vi "USO_GUI_rot_stg.vi"() -> ()   [LabVIEW 2014]
uses:
  <vilib>/Platform/TimedLoop/XDataNode/timing_clust.ctl
  <vilib>/Platform/TimedLoop/XDataNode/nitl_modes.ctl
  <vilib>/Platform/TimedLoop/XDataNode/wakeup.ctl
  gfitsio/cfitsio-bitpix.ctl
  <vilib>/platform/TimedLoop/XDataNode/XDataNode.xnode
  gfitsio/gfitsio.lvlib
  <vilib>/gmath/NI_Gmath.lvlib
  <userlib>/Newport ESP301/Newport ESP301.lvlib
  <vilib>/Platform/TimedLoop/XDataNode/XDNodeRunTimeDep.lvlib
panel:
  in  "initial absolute position":dbl=-33.5 min=-2000000000.0 max=2000000000.0 format="%.6f"
  out "Start time Array":timestamp[](array[timestamp])
  out "End time Array":timestamp[](array[timestamp])
  in  "Voltage-Retardance file path for lcvr2":path
  in  "Start observation session":bool
  out "LCVR closing\nvariable":T1(array[cluster])
  out "LCVR variable":T2
  out "Current Lcvr Temp":dbl
  out "volt set of lcvr 2":dbl[](array[numeric]) format="%_6g"
  out "volt set of lcvr 1":dbl[](array[numeric]) format="%_6g"
  in  "Voltage-Retardance file path for lcvr1":path
  in  "LCVR Set Temperature":dbl=21.0 min=10.0 max=50.0
  out "Buf no 2":bool
  out "Buf no 1":bool
  out "hout":u64
  in  "OpenStructureIn":T3={"Size"=88, "InterfaceType"=1, "Camera Number"=0, "CameraNumAtInterface"=0, "OpenFlags"=[], "OpenDWFlags"=[], "OpenPtrs"=[]} {"InterfaceType" items=["IEEE1394/FireWire", "IEEE1394/FireWire", "Matrox Helios CameraLink", "SiliconSoftware MicroEnableIII CL", "National Instruments CameraLink", "Gigabit Ethernet", "USB", "SiliconSoftware MicroEnable IV CL", "Reserved", "Reserved", "Generic CameraLink with CLSER.DLL"]}
  out "Buff_no 2":i16
  out "Buff_no1":i16
  in  "Close USO software":bool
  in  "spectroscopy/spectropolarimetry tab":enum32{"Spectroscopy", "Spectropolarimetry"}(tab) caption="Tab Control"
  in  "Slide":cluster{i32, i32}(slide)={16384, 0} scale=0.0..16400.0
  in  "Display Intensity control":bool
  in  "Control Pannel":T4
  in  "Cam Exp (msec)":dbl
  out "Cam Delay (msec)":dbl
  in  "Rot in deg":dbl min=-6000.0 max=6000.0 step=0.01
  in  "Scan steps":dbl=240.0
  out "Steps performed":i32(slide) max=190 scale=0.0..240.0
  in  "Start Spectroscopy":bool
  in  "Stop Spectroscopy":bool
  out "CCD Display":i32[][](graph)
  out "Data is stored in the folder.........":path
  in  "accept intensity":bool
  in  "Averaging \nNum":dbl=1.0
  in  "Image averaging":enum32{"Per scan", "Per Polarisation"}(radio)
  in  "LCVR Temperature in deg C\n      Set         Current":dbl[](array[numeric]) min=0.0 max=50.0
  in  "Slide sp":cluster{i32, i32}(slide)={16384, 0} scale=0.0..16400.0
  in  "accept intensity sp":bool
  out "Data is stored in the folder sp.........":path
  out "CCD Display sp":i32[][](graph)
  in  "Stop Spectroscopy sp":bool
  in  "Start Spectroscopy sp":bool
  out "Steps performed sp":i32(slide) max=190 scale=0.0..240.0
  in  "Scan steps sp":dbl=240.0
  in  "Rot in deg sp":dbl min=-6000.0 max=6000.0 step=0.01
  out "Cam Delay (msec) sp":dbl
  in  "Cam Exp (msec) sp":dbl
  in  "Display Intensity control sp":bool
  in  "Control Pannel sp":T4
  out "Motor Variable":T5={"VISA resource name"="", "Axis 2"=1, "Rotate in deg 2"=100.0, "Error In"={"status"=FALSE, "code"=0, "source"=""}}
  out "Cam Variable":T6
  in  "Rotate in deg":dbl=0.003
  in  "VISA Refnum in":refnum<visa-resource-name>
  in  "Axis":u32=1
  in  "CONTROLLER Number":string="1"
  out "Status":string
  in  "Apply":bool
  in  "InterfaceType":u32(ring)=6 items=["Ethernet"=5, "USB"=6]
  in  "Finish":bool
  out "Cam Detail":T7
  in  "Delay in msec":u32 max=4233600000
  in  "Exposure in msec":u32=30 min=500 max=4233600000
  in  "Initialise Device":u16(ring)=3 items=["Camera", "Liquid crystal", "Scan mirror", "--FF--"]
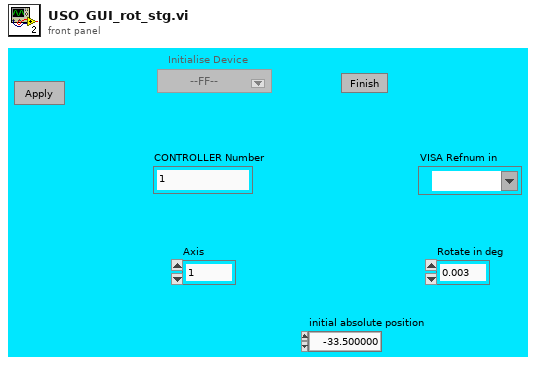
[diagram p1: front panel]
types:
  T1 = cluster{"Device Handle":u32, "Pipe 0 Handle":u32, "Pipe 1 Handle":u32}[]
  T2 = cluster{"Open USB I/O Stuff":cluster{"Device Handle":u32, "Pipe 0 Handle":u32, "Pipe 1 Handle":u32}, "volt set of lcvr 1":dbl[], "volt set of lcvr 2":dbl[], "LCVR Set Temperature":dbl, "Current Lcvr Temp":dbl}
  T3 = cluster{"Size":u16, "InterfaceType":u16, "Camera Number":u16, "CameraNumAtInterface":u16, "OpenFlags":u16[], "OpenDWFlags":u32[], "OpenPtrs":u32[]}
  T4 = cluster{"Move mirror":bool, "Preview":bool, "reset motor":bool, "motor home":bool, "Restore default values":bool}
  T5 = cluster{"VISA resource name":refnum<visa-resource-name>, "Axis 2":u32, "Rotate in deg 2":dbl, "Error In":errorcluster}
  T6 = cluster{"hout":u64, "ErrorOut":errorcluster, "Description":cluster{"Size":u16, "SensorTypeDESC":u16, "SensorSubtypeDESC":u16, "MaxHorizontalResStdDESC":u16, "MaxVerticalResStdDESC":u16, "MaxHorizontalResExtDESC":u16, "MaxVerticalResExtDESC":u16, "DynResDESC":u16, "MaxBinHorzDESC":u16, "BinHorzStepDESC":bool, "MaxBinVertDESC":u16, "BinVertStepDESC":bool, "ROIHorzStepDESC":u16, "ROIVertStepDESC":u16, "NumADCDESC":u16, "IRDESC":bool, "MinDelayDESC":u32, "MaxDelayDESC":u32, "MinDelayStepDESC":u32, "MinExpoDESC":u32, "MaxExpoDESC":u32, "MinExpoStepDESC":u32, "MinDelayIRDESC":u32, "MaxDelayIRDESC":u32, "MinExpoIRDESC":u32, "MaxExpoIRDESC":u32, "TimeTableDESC":bool, "DoubleImageDESC":bool, "MinCoolSetDESC":i16, "MaxCoolSetDESC":i16, "MDefaultCoolSetDESC":i16, "PowerDownModeDESC":bool, "OffsetRegDESC":bool, "ColorPattern":cluster{"UpperLeftColor":u8, "UpperRightColor":u8, "LowerLeftColor":u8, "LowerRightColor":u8}, "PatternTypeDESC":bool, "PixelRates":u32[], "CoversionFactors":u16[], "Reserved":u32[], "NoiseFilterCapable":bool, "HotPixelCapable":bool, "HotPixelWithNoiseFilter":bool, "ASCIITimeCapable":bool, "Extended Description":bool, "Get Extended":bool, "Reserved Flag 1":bool, "Reserved Flag 2":bool}}
  T7 = cluster{"Size":u16, "SensorTypeDESC":u16, "SensorSubtypeDESC":u16, "MaxHorizontalResStdDESC":u16, "MaxVerticalResStdDESC":u16, "MaxHorizontalResExtDESC":u16, "MaxVerticalResExtDESC":u16, "DynResDESC":u16, "MaxBinHorzDESC":u16, "BinHorzStepDESC":bool, "MaxBinVertDESC":u16, "BinVertStepDESC":bool, "ROIHorzStepDESC":u16, "ROIVertStepDESC":u16, "NumADCDESC":u16, "IRDESC":bool, "MinDelayDESC":u32, "MaxDelayDESC":u32, "MinDelayStepDESC":u32, "MinExpoDESC":u32, "MaxExpoDESC":u32, "MinExpoStepDESC":u32, "MinDelayIRDESC":u32, "MaxDelayIRDESC":u32, "MinExpoIRDESC":u32, "MaxExpoIRDESC":u32, "TimeTableDESC":bool, "DoubleImageDESC":bool, "MinCoolSetDESC":i16, "MaxCoolSetDESC":i16, "MDefaultCoolSetDESC":i16, "PowerDownModeDESC":bool, "OffsetRegDESC":bool, "ColorPattern":cluster{"UpperLeftColor":u8, "UpperRightColor":u8, "LowerLeftColor":u8, "LowerRightColor":u8}, "PatternTypeDESC":bool, "PixelRates":u32[], "CoversionFactors":u16[], "Reserved":u32[], "NoiseFilterCapable":bool, "HotPixelCapable":bool, "HotPixelWithNoiseFilter":bool, "ASCIITimeCapable":bool, "Extended Description":bool, "Get Extended":bool, "Reserved Flag 1":bool, "Reserved Flag 2":bool}
  T8 = enum16{"Find +0 Position Count", "Find Home and Index Signals", "Find Home Signal", "Find Positive Limit Signal", "Find Negative Limit Signal", "Find Positve Limit and Index Signals", "Find Negative Limit and Index Signals"}
  T9 = typedef "XDNodeRunTimeDep.lvlib/timing_clust.ctl" = cluster{"Expected End [f-1]":u64, "Actual End [f-1]":u64, "Finished Late? [f-1]":bool, "Expected End [i-1]":u64, "Actual End [i-1]":u64, "Finished Late? [i-1]":bool, "Expected Start [i]":u64, "Actual Start [i]":u64, "Expected Start [f]":u64, "Actual Start [f]":u64, "Source Name":string, "Structure Name":string, "Period":i64, "Deadline":i64, "Offset":i64, "Start":i64, "Priority":i32, "Timeout":i32, "Mode":T10, "Wakeup Reason":T11, "Error":errorcluster, "Source Type":string, "Secondary Source Type":string, "Global End Time":u64, "Global Start Time":u64, "Frame Duration":u64, "Iteration Duration":u64, "Assigned CPU":i32, "I/O Scan Engine Mode":u32}
  T10 = typedef "XDNodeRunTimeDep.lvlib/nitl_modes.ctl" = enum32{"No Change", "Process missed periods, maintain original phase", "Discard missed periods, maintain original phase", "Process missed periods, ignore original phase", "Discard missed periods, ignore original phase"}
  T11 = typedef "XDNodeRunTimeDep.lvlib/wakeup.ctl" = enum32{"Normal", "Aborted", "Asynchronous wakeup", "Timing source error", "Timed loop error", "Timeout"}
  T12 = enum8{"Enabled", "Disabled", "Disabled and Grayed Out"}
  T13 = enum16{"open", "open or create", "create or replace", "create", "open (read only)"}
  T14 = cluster{"Device Handle":u32, "Pipe 0 Handle":u32, "Pipe 1 Handle":u32}
  T15 = cluster{"Open USB I/O Stuff":cluster{"Device Handle":u32, "Pipe 0 Handle":u32, "Pipe 1 Handle":u32}, "yi":dbl[], "yi":dbl[], dbl, "Temp":dbl}
  T16 = cluster{"VISA resource name out":refnum<visa-resource-name>, "Axis":u32, "Rotate in deg":dbl, "error out":errorcluster}
  T17 = cluster{"hout":u64, "error out":errorcluster, "Description":cluster{"Size":u16, "SensorTypeDESC":u16, "SensorSubtypeDESC":u16, "MaxHorizontalResStdDESC":u16, "MaxVerticalResStdDESC":u16, "MaxHorizontalResExtDESC":u16, "MaxVerticalResExtDESC":u16, "DynResDESC":u16, "MaxBinHorzDESC":u16, "BinHorzStepDESC":bool, "MaxBinVertDESC":u16, "BinVertStepDESC":bool, "ROIHorzStepDESC":u16, "ROIVertStepDESC":u16, "NumADCDESC":u16, "IRDESC":bool, "MinDelayDESC":u32, "MaxDelayDESC":u32, "MinDelayStepDESC":u32, "MinExpoDESC":u32, "MaxExpoDESC":u32, "MinExpoStepDESC":u32, "MinDelayIRDESC":u32, "MaxDelayIRDESC":u32, "MinExpoIRDESC":u32, "MaxExpoIRDESC":u32, "TimeTableDESC":bool, "DoubleImageDESC":bool, "MinCoolSetDESC":i16, "MaxCoolSetDESC":i16, "MDefaultCoolSetDESC":i16, "PowerDownModeDESC":bool, "OffsetRegDESC":bool, "ColorPattern":cluster{"UpperLeftColor":u8, "UpperRightColor":u8, "LowerLeftColor":u8, "LowerRightColor":u8}, "PatternTypeDESC":bool, "PixelRates":u32[], "CoversionFactors":u16[], "Reserved":u32[], "NoiseFilterCapable":bool, "HotPixelCapable":bool, "HotPixelWithNoiseFilter":bool, "ASCIITimeCapable":bool, "Extended Description":bool, "Get Extended":bool, "Reserved Flag 1":bool, "Reserved Flag 2":bool}}
  T18 = typedef "gfitsio.lvlib/cfitsio-bitpix.ctl" = i32
  T19 = typedef "gfitsio.lvlib/gfitsio-refnum.ctl" = refnum<k1>
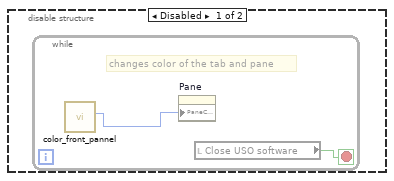
[diagram p2: hidden frame]
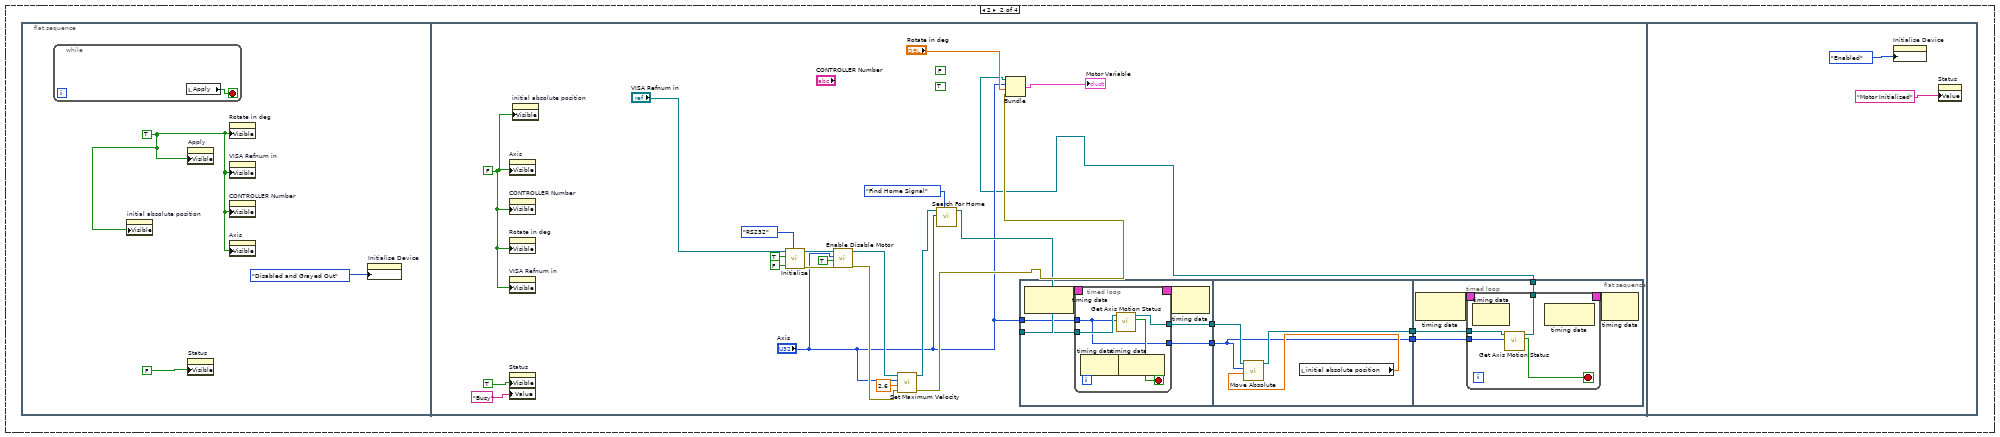
[diagram p9: hidden frame]
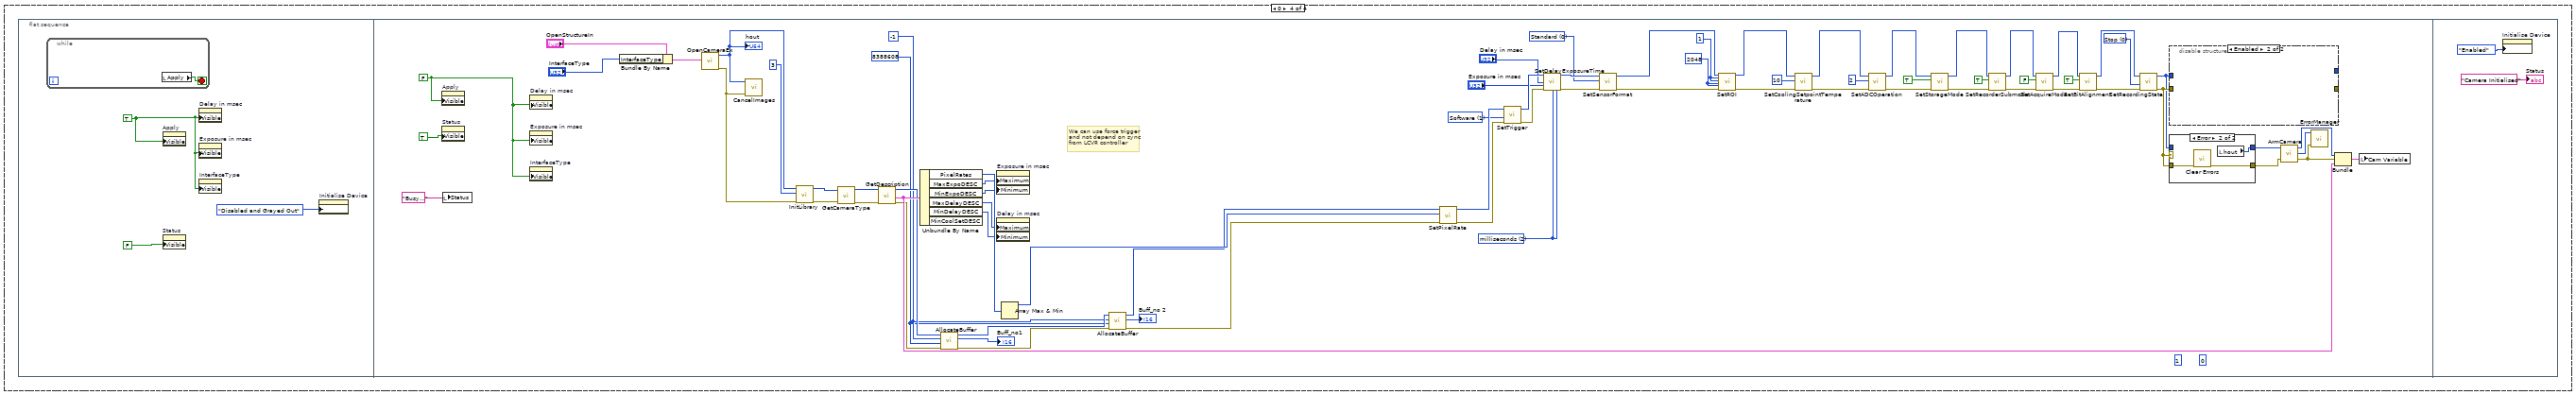
[diagram p11: hidden frame]
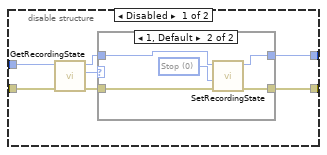
[diagram p12: hidden frame]
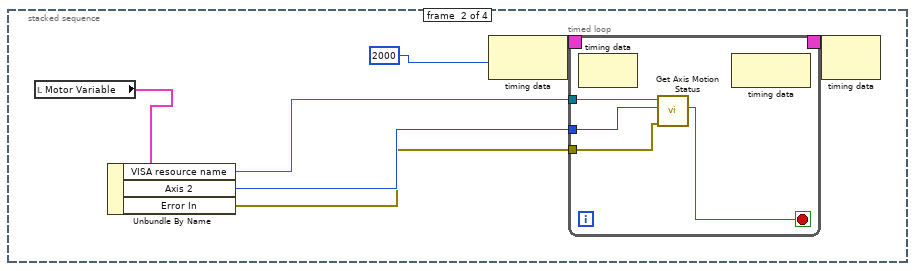
[diagram p15: hidden frame]
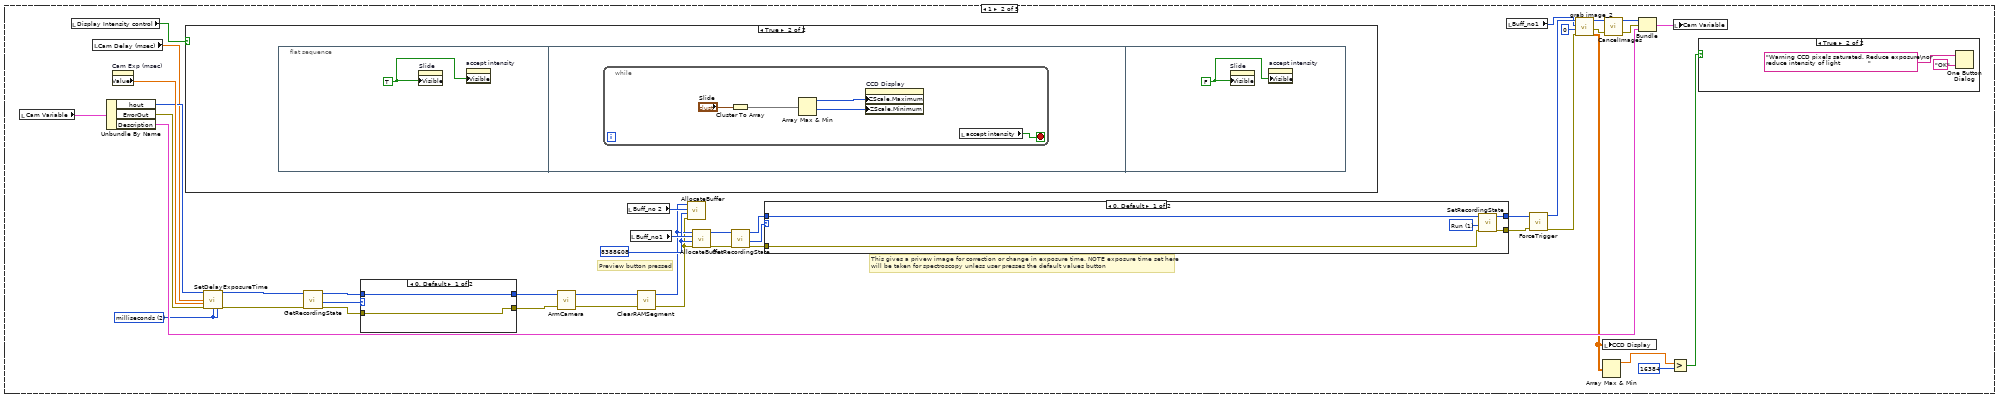
[diagram p18: hidden frame]
diagram:
  w2 = TRUE
  w3 = 2048.0 ("X Scale.Range:Maximum")
  w4 = 1.0 ("X Scale.Range:Minimum")
  w1 = FALSE
  # "Frame 0:- Initialize camera, lcvr, rotation stage\nFrame 1:- wait for rotation stage to complete roration (This is jst a safty measure, the code by default goes to frame 1 after completly initializing all components in frame 0 \n                  but a redundant frame is used for rotation stage jst to ensure completion of rotation stage's initialization)\nFrame 2:- The entire code runs in frame 2 right from previews, motor moves, frame recording, intensity range variation of image display,polcal, flat field  etc\nFrame 3:- Closes camera and LCVR and brings motor to home position and switches off the motor"
  n1 = disable-structure shown="Enabled" {
    frame Disabled {
      n2 = while {
        stop <- w6 stop-if-true
        # "changes color of the tab and pane"
        n3 = call "color_front_pannel.vi"() -> ("Resolved Color"=w5:u32)  [unwired: 11 in]
        n4 = property on="Pane" class="Pane"("PaneColor"=w5) -> ()  [unwired: 2 in, 2 out]
        n5 = local read "Close USO software"() -> (w6:bool)
      }
    }
    frame Enabled {
    }
  }
  n6 = stacked-sequence {
    frame #0 {
      n7 = Two Button Dialog(message="Initialise Devices ?", 1:"No" ("F button name (\"Cancel\")"), 2:"Yes" ("T button name (\"OK\")")) -> (T button?=w7:bool)
      n8 = case shown="True" w7 {
        frame False {
          n9 = flat-sequence {
            frame #0 {
              w11 = TRUE
              n10 = property on="Voltage-Retardance file path for lcvr2" class="Path"("Visible"=w11) -> ()  [unwired: 2 in, 2 out]
              n11 = property on="Voltage-Retardance file path for lcvr1" class="Path"("Visible"=w11) -> ()  [unwired: 2 in, 2 out]
              n12 = property on="initial absolute position" class="DigNum (strict)"("Visible"=w11) -> ()  [unwired: 2 in, 2 out]
              n13 = while {
                stop <- w12 stop-if-true
                n14 = local read "Apply"() -> (w12:bool)
              }
              n15 = property on="Apply" class="Bool (strict)"("Visible"=w11) -> ()  [unwired: 2 in, 2 out]
            }
            frame #1 {
              w17 = 1 ("Axis (1)")
              w14 = FALSE
              w52 = 21.0
              w69 = u32 8388608 ("Size")
              w70 = i16 -1 ("BufNr")
              w77 = u16 0 items=["Stop", "Run"] ("RecordingState")
              # "Dont use Arm Cam.vi here coz the camera FPGA \"remembers\"\nthe settings that were used in its previous use. So the camera \nwill be initialized to those settings automatically"
              # "As the user has not selected device initilization, all devices will be initiated to their default value"
              n16 = local read "Voltage-Retardance file path for lcvr2"() -> (w38:path)
              n17 = local read "Voltage-Retardance file path for lcvr1"() -> (w39:path)
              n18 = property on="Apply" class="Bool (strict)"("Visible"=w14) -> ()  [unwired: 2 in, 2 out]
              n19 = property on="Voltage-Retardance file path for lcvr2" class="Path"("Visible"=w14) -> ()  [unwired: 2 in, 2 out]
              n20 = property on="initial absolute position" class="DigNum (strict)"("Visible"=w14) -> ()  [unwired: 2 in, 2 out]
              n21 = property on="Voltage-Retardance file path for lcvr1" class="Path"("Visible"=w14) -> ()  [unwired: 2 in, 2 out]
              n22 = call "Meadowlark USB Easy Open.vi"() -> ("USB Device and Pipes Array"=w47:T1, "Device Count"=w13:u32)  [unwired: 1 out]
              n23 = case shown="0" w13 {
                frame 0 {
                  n24 = One Button Dialog(message="WARNING !!\nNO LCVR'S DETECTED", button name ("OK")="OK") -> ()  [unwired: 1 out]
                }
                frame 1, Default {
                }
              }
              n25 = call "volt vs retardance.vi"("file path (dialog if empty)"=w38) -> ("retardance in degree(known)"=w40:dbl[], "Voltage(unknown)"=w41:dbl[])  [unwired: 9 in]
              n26 = local write "LCVR closing\nvariable"(w47) -> ()
              n27 = local read "OpenStructureIn"() -> (w64:T3)
              n28 = call "volt vs retardance.vi"("file path (dialog if empty)"=w39) -> ("retardance in degree(known)"=w57:dbl[], "Voltage(unknown)"=w56:dbl[])  [unwired: 9 in]
              n29 = Index Array(array=w47, index=0) -> (element=w53:T14)
              n30 = local read "VISA Refnum in"() -> (w37:refnum<visa-resource-name>)
              n31 = local read "InterfaceType"() -> (w62:u32)
              n32 = call "Set temp.vi"("Temp"=w52, "USB Open Device Cluster"=w53) -> ()  [unwired: 1 in]
              n33 = call <vilib>:"Spline Interpolation 1D.vi"("xi"=dbl[] [45.0, 135.0, 135.0, 225.0], "X"=w57, "Y"=w56) -> ("yi"=w50:dbl[])  [unwired: 6 in, 2 out]
              n34 = call "read temp.vi"("USB Open Device Cluster"=w53) -> ("Temp"=w51:dbl)
              n35 = call <vilib>:"Spline Interpolation 1D.vi"("xi"=dbl[] [54.74, 125.26, 234.74, 54.74], "X"=w40, "Y"=w41) -> ("yi"=w49:dbl[])  [unwired: 6 in, 2 out]
              n36 = local write "LCVR Set Temperature"(w52) -> ()
              n37 = local write "Current Lcvr Temp"(w51) -> ()
              n38 = Bundle By Name(cluster=w64, "InterfaceType"=w62) -> (w61:T3)
              n39 = local write "volt set of lcvr 1"(w50) -> ()
              n40 = local write "volt set of lcvr 2"(w49) -> ()
              n41 = Bundle("Open USB I/O Stuff"=w53, "yi"=w50, "yi"=w49, w52, "Temp"=w51) -> (w48:T15)  [unwired: 1 in]
              n42 = local write "LCVR variable"(w48) -> ()
              n43 = call <userlib>:"OpenCameraEx.vi"("OpenStructureIn"=w61) -> ("error out"=w59:errorcluster, "hout"=w60:u64)  [unwired: 3 in, 2 out]
              n44 = call <userlib>:"CancelImages.vi"("error in (no error)"=w59, "ph"=w60) -> ()  [unwired: 1 in, 3 out]
              n45 = call <userlib>:"Initialize.vi"("VISA resource name"=w37, "ID Query (True)"=TRUE, "Reset (False)"=FALSE, "Serial Link (RS232)"=enum16{"RS232", "USB"}."RS232") -> ("VISA resource name out"=w33:refnum<visa-resource-name>, "error out"=w31:errorcluster)  [unwired: 5 in]
              n46 = call <userlib>:"InitLibrary.vi"("error in (no error)"=w59, "InterfaceType"=u32 3, "ph"=w60) -> ("error out"=w83:errorcluster, "hout"=w84:u64)  [unwired: 7 in]
              n47 = local read "Rotate in deg"() -> (w78:dbl)
              n48 = call <userlib>:"GetCameraType.vi"("ph"=w84, "error in (no error)"=w83) -> ("hout"=w82:u64, "error out"=w81:errorcluster)  [unwired: 1 in, 2 out]
              n49 = local read "Axis"() -> (w30:u32)
              n50 = call <userlib>:"Enable Disable Motor.vi"("error in (no error)"=w31, "Action (F - OFF)"=TRUE, "Axis (1)"=w17, "VISA resource name"=w33) -> ("error out"=w24:errorcluster, "VISA resource name out"=w26:refnum<visa-resource-name>)  [unwired: 2 in]
              n51 = call <userlib>:"GetDescription.vi"("ErrorIn"=w81, "ph"=w82) -> ("ErrorOut"=w43:errorcluster, "Description"=w80:T7, "hout"=w45:u64)  [unwired: 2 in, 1 out]
              n52 = local write "Cam Detail"(w80) -> ()
              n53 = call <userlib>:"Set Maximum Velocity.vi"("error in (no error)"=w24, "Maximum Velocity (0 units/s)"=2.6, "Axis (1)"=w17, "VISA resource name"=w26) -> ("error out"=w22:errorcluster, "VISA resource name out"=w23:refnum<visa-resource-name>)  [unwired: 2 in]
              n54 = call <userlib>:"SetBitAlignment.vi"("error in (no error)"=w43, "BitAlignent"=TRUE, "ph"=w45) -> ("error out"=w42:errorcluster, "hout"=w44:u64)  [unwired: 2 in, 1 out]
              n55 = call <userlib>:"Search For Home.vi"("Home mode"=T8."Find Home Signal", "error in (no error)"=w22, "Axis (1)"=w17, "VISA resource name"=w23) -> ("error out"=w27:errorcluster, "VISA resource name out"=w16:refnum<visa-resource-name>)  [unwired: 3 in]
              n56 = Bundle("VISA resource name out"=w15, "Axis"=w30, "Rotate in deg"=w78, "error out"=w27) -> (w29:T16)  [unwired: 1 in]
              n57 = call <userlib>:"SetRecordingState.vi"("ErrorIn"=w42, "RecordingState"=w77, "ph"=w44) -> ("ErrorOut"=w65:errorcluster, "hout"=w66:u64)  [unwired: 2 in, 1 out]
              n58 = call <userlib>:"ErrorManager.vi"("ErrorIn"=w65, "ErrorCode"=w66) -> ()  [unwired: 3 in, 1 out]
              n59 = flat-sequence {
                tunnel: w16 -> [w90]
                tunnel: w17 -> [w89]
                tunnel: [w88] -> w21
                tunnel: [w87] -> w20
                tunnel: w21 -> [w104]
                tunnel: w20 -> [w101]
                tunnel: [w102] -> w19
                tunnel: [w101] -> w18
                tunnel: w19 -> [w107]
                tunnel: w18 -> [w106]
                tunnel: [w105] -> w15
                frame #0 {
                  n60 = node-c288() -> (w92:T9)  [unwired: 1 in]
                  n61 = timed-loop {
                    timing: w92 -> [_]
                    timing-out: [_] -> w91
                    tunnel: w90 -> [w96]
                    tunnel: w89 -> [w93]
                    tunnel: [w95] -> w88
                    tunnel: [w93] -> w87
                    stop <- w94 stop-if-true
                    n62 = node-c288() -> ()  [unwired: 1 in, 1 out]
                    n63 = node-c288() -> ()  [unwired: 1 in, 1 out]
                    n64 = call <userlib>:"Get Axis Motion Status.vi"("Axis (1)"=w93, "VISA resource name"=w96) -> ("Motion Done"=w94:bool, "VISA resource name out"=w95:refnum<visa-resource-name>)  [unwired: 3 in, 1 out]
                  }
                  n65 = node-c288(w91) -> ()  [unwired: 1 out]
                }
                frame #1 {
                  n66 = local read "initial absolute position"() -> (w103:dbl)
                  n67 = call <userlib>:"Move Absolute.vi"("Position (0 units)"=w103, "Axis (1)"=w101, "VISA resource name"=w104) -> ("VISA resource name out"=w102:refnum<visa-resource-name>)  [unwired: 3 in, 1 out]
                }
                frame #2 {
                  n68 = node-c288() -> (w109:T9)  [unwired: 1 in]
                  n69 = timed-loop {
                    timing: w109 -> [_]
                    timing-out: [_] -> w108
                    tunnel: w107 -> [w113]
                    tunnel: w106 -> [w112]
                    tunnel: [w111] -> w105
                    stop <- w110 stop-if-true
                    n70 = node-c288() -> ()  [unwired: 1 in, 1 out]
                    n71 = call <userlib>:"Get Axis Motion Status.vi"("Axis (1)"=w112, "VISA resource name"=w113) -> ("Motion Done"=w110:bool, "VISA resource name out"=w111:refnum<visa-resource-name>)  [unwired: 3 in, 1 out]
                    n72 = node-c288() -> ()  [unwired: 1 in, 1 out]
                  }
                  n73 = node-c288(w108) -> ()  [unwired: 1 out]
                }
              }
              n74 = case shown="Error" w65 {
                tunnel: [w119 w121] -> w73
                tunnel: w65 -> [w119 w122]
                tunnel: w66 -> [w118 _]
                tunnel: [w118 w120] -> w76
                tunnel: w45 -> [_ w120]
                frame No Error {
                }
                frame Error {
                  n75 = call <vilib>:"Clear Errors.vi"("error in (no error)"=w122) -> ("error out"=w121:errorcluster)  [unwired: 5 in, 1 out]
                }
              }
              n76 = local write "Motor Variable"(w29) -> ()
              n77 = call <userlib>:"AllocateBuffer.vi"("error in (no error)"=w73, "Size"=w69, "BufNr"=w70, "ph"=w76) -> ("error out"=w72:errorcluster, "BufNrOut"=w68:i16, "hout"=w75:u64)  [unwired: 2 in, 3 out]
              n78 = local write "Buff_no1"(w68) -> ()
              n79 = call <userlib>:"AllocateBuffer.vi"("error in (no error)"=w72, "Size"=w69, "BufNr"=w70, "ph"=w75) -> ("error out"=w71:errorcluster, "BufNrOut"=w67:i16, "hout"=w74:u64)  [unwired: 2 in, 3 out]
              n80 = Bundle("hout"=w74, "error out"=w71, "Description"=w80) -> (→"Cam Variable":T17)  [unwired: 1 in]
              n81 = local write "Buff_no 2"(w67) -> ()
            }
          }
        }
        frame True {
          n82 = flat-sequence {
            frame #0 {
              w124 = TRUE
              n83 = property on="Finish" class="Bool"("Visible"=w124) -> ()  [unwired: 2 in, 2 out]
              n84 = property on="Initialise Device" class="Ring (strict)"("DisabledEnum"=T12."Enabled" ("Disabled")) -> ()  [unwired: 2 in, 2 out]
              n85 = property on="Initialise Device" class="Ring (strict)"("Visible"=w124) -> ()  [unwired: 2 in, 2 out]
            }
            frame #1 {
              n86 = while {
                stop <- w126 stop-if-true
                n87 = event shown="[0] \"Finish\", \"Initialise Device\": Value Change" {
                  selector: _ -> [_]
                  dyn-events: _ -> [_]
                  timeout: _ -> [_]
                  tunnel: ["Finish"] -> w126
                  tunnel: [w128] -> w125
                  event "Finish", "Initialise Device": Value Change {
                    n88 = event-data() -> ()  [unwired: 1 in, 1 out]
                    n89 = case shown="True" "Finish" {
                      tunnel: [w130 3] -> w128
                      tunnel: "Initialise Device" -> [w130 _]
                      frame False {
                      }
                      frame True {
                      }
                    }
                  }
                }
                n90 = case shown="1" w125 {
                  frame 1 {
                    n91 = flat-sequence {
                      frame #0 {
                        w132 = TRUE ("Visible")
                        n92 = while {
                          stop <- w136 stop-if-true
                          n93 = local read "Apply"() -> (w136:bool)
                        }
                        n94 = property on="Voltage-Retardance file path for lcvr2" class="Path"("Visible"=w132) -> ()  [unwired: 2 in, 2 out]
                        n95 = property on="Apply" class="Bool (strict)"("Visible"=TRUE) -> ()  [unwired: 2 in, 2 out]
                        n96 = property on="Voltage-Retardance file path for lcvr1" class="Path"("Visible"=w132) -> ()  [unwired: 2 in, 2 out]
                        n97 = property on="LCVR Set Temperature" class="DigNum (strict)"("Visible"=w132) -> ()  [unwired: 2 in, 2 out]
                        n98 = property on="Status" class="Str"("Visible"=FALSE) -> ()  [unwired: 2 in, 2 out]
                        n99 = property on="Initialise Device" class="Ring (strict)"("DisabledEnum"=T12."Disabled and Grayed Out" ("Disabled")) -> ()  [unwired: 2 in, 2 out]
                      }
                      frame #1 {
                        w140 = FALSE ("Visible")
                        n100 = property on="Apply" class="Bool (strict)"("Visible"=w140) -> ()  [unwired: 2 in, 2 out]
                        n101 = property on="Status" class="Str"("Visible"=TRUE) -> ()  [unwired: 2 in, 2 out]
                        n102 = local write "Status"("Busy...." ("Status")) -> ()
                        n103 = property on="Voltage-Retardance file path for lcvr2" class="Path"("Visible"=w140) -> ()  [unwired: 2 in, 2 out]
                        n104 = property on="Voltage-Retardance file path for lcvr1" class="Path"("Visible"=w140) -> ()  [unwired: 2 in, 2 out]
                        n105 = property on="LCVR Set Temperature" class="DigNum (strict)"("Visible"=w140) -> ()  [unwired: 2 in, 2 out]
                        n106 = call "Meadowlark USB Easy Open.vi"() -> ("USB Device and Pipes Array"=w139:T1, "Device Count"=w137:u32)  [unwired: 1 out]
                        n107 = case shown="0" w137 {
                          frame 0 {
                            n108 = One Button Dialog(message="WARNING !!\nNO LCVR'S DETECTED", button name ("OK")="OK") -> ()  [unwired: 1 out]
                          }
                          frame 1, Default {
                          }
                        }
                        n109 = local read "Current Lcvr Temp"() -> (w145:dbl)
                        n110 = local read "volt set of lcvr 1"() -> (w147:dbl[])
                        n111 = local read "volt set of lcvr 2"() -> (w148:dbl[])
                        n112 = local write "LCVR closing\nvariable"(w139) -> ()
                        n113 = call "volt vs retardance.vi"("file path (dialog if empty)"="Voltage-Retardance file path for lcvr2") -> ("retardance in degree(known)"=w142:dbl[], "Voltage(unknown)"=w143:dbl[])  [unwired: 9 in]
                        n114 = Index Array(array=w139, index=0) -> (element=w138:T14)
                        n115 = call "Set temp.vi"("Temp"="LCVR Set Temperature", "USB Open Device Cluster"=w138) -> ()  [unwired: 1 in]
                        n116 = call "read temp.vi"("USB Open Device Cluster"=w138) -> ("Temp"=→"Current Lcvr Temp":dbl)
                        n117 = Bundle("Open USB I/O Stuff"=w138, "volt set of lcvr 1"=w147, "volt set of lcvr 2"=w148, "LCVR Set Temperature"="LCVR Set Temperature", "Current Lcvr Temp"=w145) -> (w144:T2)  [unwired: 1 in]
                        n118 = call "volt vs retardance.vi"("file path (dialog if empty)"="Voltage-Retardance file path for lcvr1") -> ("retardance in degree(known)"=w158:dbl[], "Voltage(unknown)"=w157:dbl[])  [unwired: 9 in]
                        n119 = local write "LCVR variable"(w144) -> ()
                        n120 = call <vilib>:"Spline Interpolation 1D.vi"("xi"=dbl[] [45.0, 135.0, 135.0, 225.0], "X"=w158, "Y"=w157) -> ("yi"=→"volt set of lcvr 1":dbl[])  [unwired: 6 in, 2 out]
                        n121 = call <vilib>:"Spline Interpolation 1D.vi"("xi"=dbl[] [54.74, 125.26, 234.74, 54.74], "X"=w142, "Y"=w143) -> ("yi"=→"volt set of lcvr 2":dbl[])  [unwired: 6 in, 2 out]
                      }
                      frame #2 {
                        n122 = property on="Initialise Device" class="Ring (strict)"("DisabledEnum"=T12."Enabled" ("Disabled")) -> ()  [unwired: 2 in, 2 out]
                        n123 = local write "Status"("LCVR Initialised" ("Status")) -> ()
                      }
                    }
                  }
                  frame 2 {
                    n124 = flat-sequence {
                      frame #0 {
                        w164 = TRUE
                        n125 = while {
                          stop <- w167 stop-if-true
                          n126 = local read "Apply"() -> (w167:bool)
                        }
                        n127 = property on="initial absolute position" class="DigNum (strict)"("Visible"=w164) -> ()  [unwired: 2 in, 2 out]
                        n128 = property on="Apply" class="Bool (strict)"("Visible"=w164) -> ()  [unwired: 2 in, 2 out]
                        n129 = property on="Status" class="Str"("Visible"=FALSE) -> ()  [unwired: 2 in, 2 out]
                        n130 = property on="Rotate in deg" class="DigNum (strict)"("Visible"=w164) -> ()  [unwired: 2 in, 2 out]
                        n131 = property on="VISA Refnum in" class="VISAName"("Visible"=w164) -> ()  [unwired: 2 in, 2 out]
                        n132 = property on="CONTROLLER Number" class="Str"("Visible"=w164) -> ()  [unwired: 2 in, 2 out]
                        n133 = property on="Axis" class="DigNum (strict)"("Visible"=w164) -> ()  [unwired: 2 in, 2 out]
                        n134 = property on="Initialise Device" class="Ring (strict)"("DisabledEnum"=T12."Disabled and Grayed Out" ("Disabled")) -> ()  [unwired: 2 in, 2 out]
                      }
                      frame #1 {
                        w175 = FALSE
                        (unwired) TRUE ("MOTOR OFF/ON")
                        (unwired) FALSE ("MODE")
                        n135 = property on="Axis" class="DigNum (strict)"("Visible"=w175) -> ()  [unwired: 2 in, 2 out]
                        n136 = property on="CONTROLLER Number" class="Str"("Visible"=w175) -> ()  [unwired: 2 in, 2 out]
                        n137 = property on="Rotate in deg" class="DigNum (strict)"("Visible"=w175) -> ()  [unwired: 2 in, 2 out]
                        n138 = property on="VISA Refnum in" class="VISAName"("Visible"=w175) -> ()  [unwired: 2 in, 2 out]
                        n139 = property on="Status" class="Str"("Visible"=TRUE, "Value"="Busy") -> ()  [unwired: 2 in, 2 out]
                        n140 = property on="initial absolute position" class="DigNum (strict)"("Visible"=w175) -> ()  [unwired: 2 in, 2 out]
                        n141 = call <userlib>:"Initialize.vi"("VISA resource name"="VISA Refnum in", "ID Query (True)"=TRUE, "Reset (False)"=FALSE, "Serial Link (RS232)"=enum16{"RS232", "USB"}."RS232") -> ("VISA resource name out"=w185:refnum<visa-resource-name>, "error out"=w184:errorcluster)  [unwired: 5 in]
                        n142 = call <userlib>:"Enable Disable Motor.vi"("error in (no error)"=w184, "Action (F - OFF)"=TRUE, "Axis (1)"="Axis", "VISA resource name"=w185) -> ("error out"=w179:errorcluster, "VISA resource name out"=w181:refnum<visa-resource-name>)  [unwired: 2 in]
                        n143 = call <userlib>:"Set Maximum Velocity.vi"("error in (no error)"=w179, "Maximum Velocity (0 units/s)"=2.6, "Axis (1)"="Axis", "VISA resource name"=w181) -> ("error out"=w178:errorcluster, "VISA resource name out"=w177:refnum<visa-resource-name>)  [unwired: 2 in]
                        n144 = call <userlib>:"Search For Home.vi"("Home mode"=T8."Find Home Signal", "Axis (1)"="Axis", "VISA resource name"=w177) -> ("VISA resource name out"=w174:refnum<visa-resource-name>)  [unwired: 4 in, 1 out]
                        n145 = Bundle("VISA resource name out"=w168, "Axis"="Axis", "Rotate in deg"="Rotate in deg", "error out"=w178) -> (→"Motor Variable":T16)  [unwired: 1 in]
                        n146 = flat-sequence {
                          tunnel: w174 -> [w196]
                          tunnel: "Axis" -> [w195]
                          tunnel: [w194] -> w172
                          tunnel: [w193] -> w171
                          tunnel: w172 -> [w210]
                          tunnel: w171 -> [w207]
                          tunnel: [w208] -> w170
                          tunnel: [w207] -> w169
                          tunnel: w170 -> [w213]
                          tunnel: w169 -> [w212]
                          tunnel: [w211] -> w168
                          frame #0 {
                            n147 = node-c288() -> (w198:T9)  [unwired: 1 in]
                            n148 = timed-loop {
                              timing: w198 -> [_]
                              timing-out: [_] -> w197
                              tunnel: w196 -> [w202]
                              tunnel: w195 -> [w199]
                              tunnel: [w201] -> w194
                              tunnel: [w199] -> w193
                              stop <- w200 stop-if-true
                              n149 = node-c288() -> ()  [unwired: 1 in, 1 out]
                              n150 = node-c288() -> ()  [unwired: 1 in, 1 out]
                              n151 = call <userlib>:"Get Axis Motion Status.vi"("Axis (1)"=w199, "VISA resource name"=w202) -> ("Motion Done"=w200:bool, "VISA resource name out"=w201:refnum<visa-resource-name>)  [unwired: 3 in, 1 out]
                            }
                            n152 = node-c288(w197) -> ()  [unwired: 1 out]
                          }
                          frame #1 {
                            n153 = local read "initial absolute position"() -> (w209:dbl)
                            n154 = call <userlib>:"Move Absolute.vi"("Position (0 units)"=w209, "Axis (1)"=w207, "VISA resource name"=w210) -> ("VISA resource name out"=w208:refnum<visa-resource-name>)  [unwired: 3 in, 1 out]
                          }
                          frame #2 {
                            n155 = node-c288() -> (w215:T9)  [unwired: 1 in]
                            n156 = timed-loop {
                              timing: w215 -> [_]
                              timing-out: [_] -> w214
                              tunnel: w213 -> [w219]
                              tunnel: w212 -> [w218]
                              tunnel: [w217] -> w211
                              stop <- w216 stop-if-true
                              n157 = node-c288() -> ()  [unwired: 1 in, 1 out]
                              n158 = call <userlib>:"Get Axis Motion Status.vi"("Axis (1)"=w218, "VISA resource name"=w219) -> ("Motion Done"=w216:bool, "VISA resource name out"=w217:refnum<visa-resource-name>)  [unwired: 3 in, 1 out]
                              n159 = node-c288() -> ()  [unwired: 1 in, 1 out]
                            }
                            n160 = node-c288(w214) -> ()  [unwired: 1 out]
                          }
                        }
                      }
                      frame #2 {
                        n161 = property on="Initialise Device" class="Ring (strict)"("DisabledEnum"=T12."Enabled" ("Disabled")) -> ()  [unwired: 2 in, 2 out]
                        n162 = property on="Status" class="Str"("Value"="Motor Initialized" ("Status")) -> ()  [unwired: 2 in, 2 out]
                      }
                    }
                  }
                  frame 3, Default {
                    # "This is do nothing Case. Can be used to add components for the future"
                  }
                  frame 0 {
                    n163 = flat-sequence {
                      frame #0 {
                        w227 = TRUE
                        n164 = while {
                          stop <- w229 stop-if-true
                          n165 = local read "Apply"() -> (w229:bool)
                        }
                        n166 = property on="Apply" class="Bool (strict)"("Visible"=w227) -> ()  [unwired: 2 in, 2 out]
                        n167 = property on="Status" class="Str"("Visible"=FALSE) -> ()  [unwired: 2 in, 2 out]
                        n168 = property on="Delay in msec" class="DigNum (strict)"("Visible"=w227) -> ()  [unwired: 2 in, 2 out]
                        n169 = property on="Exposure in msec" class="DigNum (strict)"("Visible"=w227) -> ()  [unwired: 2 in, 2 out]
                        n170 = property on="InterfaceType" class="Ring (strict)"("Visible"=w227) -> ()  [unwired: 2 in, 2 out]
                        n171 = property on="Initialise Device" class="Ring (strict)"("DisabledEnum"=T12."Disabled and Grayed Out" ("Disabled")) -> ()  [unwired: 2 in, 2 out]
                      }
                      frame #1 {
                        w245 = u16 0 items=["Stop", "Run"] ("RecordingState")
                        w262 = u32 8388608 ("Size")
                        w263 = i16 -1 ("BufNr")
                        w271 = FALSE
                        w275 = u16 2 items=["nanoseconds", "microseconds", "milliseconds"] ("DelayTimeBase")
                        (unwired) u32 0 ("element")
                        (unwired) u16 1 ("ActSeg")
                        w284 = u16 0 items=["Standard", "Extended"] ("SensorIn")
                        w287 = u16 2048 ("ROIX1")
                        w288 = u16 1 ("ROIX0")
                        w295 = u16 1 items=["Auto", "Software", "External sequence start ", "External exposure control"] ("TriggerMode")
                        # "We can use force trigger\nand not depend on sync\nfrom LCVR controller"
                        n172 = property on="Apply" class="Bool (strict)"("Visible"=w271) -> ()  [unwired: 2 in, 2 out]
                        n173 = property on="Status" class="Str"("Visible"=TRUE) -> ()  [unwired: 2 in, 2 out]
                        n174 = local write "Status"("Busy..." ("Status")) -> ()
                        n175 = property on="Delay in msec" class="DigNum (strict)"("Visible"=w271) -> ()  [unwired: 2 in, 2 out]
                        n176 = property on="Exposure in msec" class="DigNum (strict)"("Visible"=w271) -> ()  [unwired: 2 in, 2 out]
                        n177 = property on="InterfaceType" class="Ring (strict)"("Visible"=w271) -> ()  [unwired: 2 in, 2 out]
                        n178 = Bundle By Name(cluster="OpenStructureIn", "InterfaceType"="InterfaceType") -> (w253:T3)
                        n179 = call <userlib>:"OpenCameraEx.vi"("OpenStructureIn"=w253) -> ("error out"=w240:errorcluster, "hout"=w241:u64)  [unwired: 3 in, 2 out]
                        "hout" <- w241
                        n180 = call <userlib>:"CancelImages.vi"("error in (no error)"=w240, "ph"=w241) -> ()  [unwired: 1 in, 3 out]
                        n181 = call <userlib>:"InitLibrary.vi"("error in (no error)"=w240, "InterfaceType"=u32 3, "ph"=w241) -> ("error out"=w302:errorcluster, "hout"=w303:u64)  [unwired: 7 in]
                        n182 = call <userlib>:"GetCameraType.vi"("ph"=w303, "error in (no error)"=w302) -> ("hout"=w300:u64, "error out"=w301:errorcluster)  [unwired: 1 in, 2 out]
                        n183 = call <userlib>:"GetDescription.vi"("ErrorIn"=w301, "ph"=w300) -> ("ErrorOut"=w261:errorcluster, "Description"=w268:T7, "hout"=w265:u64)  [unwired: 2 in, 1 out]
                        n184 = Unbundle By Name(w268) -> ("PixelRates"=w299:u32[], "MaxExpoDESC"=w292:u32, "MinExpoDESC"=w291:u32, "MaxDelayDESC"=w290:u32, "MinDelayDESC"=w289:u32)  [unwired: 1 out]
                        n185 = call <userlib>:"AllocateBuffer.vi"("error in (no error)"=w261, "Size"=w262, "BufNr"=w263, "ph"=w265) -> ("error out"=w260:errorcluster, "BufNrOut"=→"Buff_no1":i16, "hout"=w264:u64)  [unwired: 2 in, 3 out]
                        n186 = property on="Exposure in msec" class="DigNum (strict)"("Maximum"=w292, "Minimum"=w291) -> ()  [unwired: 2 in, 2 out]
                        n187 = property on="Delay in msec" class="DigNum (strict)"("Maximum"=w290, "Minimum"=w289) -> ()  [unwired: 2 in, 2 out]
                        n188 = Array Max & Min(array=w299) -> (max value=w298:u32)  [unwired: 3 out]
                        n189 = call <userlib>:"AllocateBuffer.vi"("error in (no error)"=w260, "Size"=w262, "BufNr"=w263, "ph"=w264) -> ("error out"=w256:errorcluster, "BufNrOut"=→"Buff_no 2":i16, "hout"=w257:u64)  [unwired: 2 in, 3 out]
                        n190 = call <userlib>:"SetPixelRate.vi"("error in (no error)"=w256, "PixelRate"=w298, "ph"=w257) -> ("error out"=w297:errorcluster, "hout"=w296:u64)  [unwired: 2 in, 1 out]
                        n191 = call <userlib>:"SetTrigger.vi"("error in (no error)"=w297, "TriggerMode"=w295, "ph"=w296) -> ("error out"=w293:errorcluster, "hout"=w294:u64)  [unwired: 2 in, 1 out]
                        n192 = call <userlib>:"SetDelayExposureTime.vi"("ph"=w294, "Delay"="Delay in msec", "Exposure"="Exposure in msec", "error in (no error)"=w293, "DelayTimeBase"=w275, "ExposureTimeBase"=w275) -> ("hout"=w285:u64, "error out"=w286:errorcluster)  [unwired: 7 in, 1 out]
                        n193 = call <userlib>:"SetSensorFormat.vi"("ErrorIn"=w286, "SensorIn"=w284, "ph"=w285) -> ("ErrorOut"=w282:errorcluster, "hout"=w283:u32)  [unwired: 2 in, 1 out]
                        n194 = call <userlib>:"SetROI.vi"("ph"=w283, "ROIX0"=w288, "ROIY0"=w288, "ROIX1"=w287, "ROIY1"=w287, "error in (no error)"=w282) -> ("hout"=w280:u64, "error out"=w281:errorcluster)  [unwired: 12 in]
                        n195 = call <userlib>:"SetCoolingSetpointTemperature.vi"("error in (no error)"=w281, "CoolSet"=i16 10, "ph"=w280) -> ("error out"=w279:errorcluster, "hout"=w278:u64)  [unwired: 2 in, 1 out]
                        n196 = call <userlib>:"SetADCOperation.vi"("error in (no error)"=w279, "ADCOperation"=u16 2, "ph"=w278) -> ("error out"=w250:errorcluster, "hout"=w251:u64)  [unwired: 2 in, 1 out]
                        n197 = call <userlib>:"SetStorageMode.vi"("error in (no error)"=w250, "StorageMode"=TRUE, "ph"=w251) -> ("error out"=w237:errorcluster, "hout"=w239:u64)  [unwired: 2 in, 1 out]
                        n198 = call <userlib>:"SetRecorderSubmode.vi"("error in (no error)"=w237, "RecorderSubMode"=TRUE, "ph"=w239) -> ("error out"=w236:errorcluster, "hout"=w238:u64)  [unwired: 2 in, 1 out]
                        n199 = call <userlib>:"SetAcquireMode.vi"("error in (no error)"=w236, "UseAcquireEnable"=FALSE, "ph"=w238) -> ("error out"=w232:errorcluster, "hout"=w234:u64)  [unwired: 2 in, 1 out]
                        n200 = call <userlib>:"SetBitAlignment.vi"("error in (no error)"=w232, "BitAlignent"=TRUE, "ph"=w234) -> ("error out"=w231:errorcluster, "hout"=w233:u64)  [unwired: 2 in, 1 out]
                        n201 = call <userlib>:"SetRecordingState.vi"("ErrorIn"=w231, "RecordingState"=w245, "ph"=w233) -> ("ErrorOut"=w247:errorcluster, "hout"=w246:u64)  [unwired: 2 in, 1 out]
                        n202 = disable-structure shown="Enabled" {
                          disable-tunnel: [w307 _] -> _
                          disable-tunnel: [w306 _] -> _
                          disable-tunnel: w247 -> [w305 _]
                          disable-tunnel: w246 -> [w304 _]
                          frame Disabled {
                            n203 = call <userlib>:"GetRecordingState.vi"("ErrorIn"=w305, "ph"=w304) -> ("ErrorOut"=w310:errorcluster, "Error"=w308:i32, "hout"=w309:u64)  [unwired: 2 in, 1 out]
                            n204 = case shown="1, Default" w308 {
                              tunnel: [w312 w316] -> w307
                              tunnel: [w311 w315] -> w306
                              tunnel: w310 -> [w311 w314]
                              tunnel: w309 -> [w312 w313]
                              frame 0 {
                              }
                              frame 1, Default {
                                w317 = u16 0 items=["Stop", "Run"] ("RecordingState")
                                n205 = call <userlib>:"SetRecordingState.vi"("ErrorIn"=w314, "RecordingState"=w317, "ph"=w313) -> ("ErrorOut"=w315:errorcluster, "hout"=w316:u64)  [unwired: 2 in, 1 out]
                              }
                            }
                          }
                          frame Enabled {
                          }
                        }
                        n206 = case shown="Error" w247 {
                          tunnel: w246 -> [w318 _]
                          tunnel: [w319 w321] -> w243
                          tunnel: w247 -> [w319 w322]
                          tunnel: [w318 w320] -> w244
                          frame No Error {
                          }
                          frame Error {
                            n207 = call <vilib>:"Clear Errors.vi"("error in (no error)"=w322) -> ("error out"=w321:errorcluster)  [unwired: 5 in, 1 out]
                            n208 = local read "hout"() -> (w320:u64)
                          }
                        }
                        n209 = call <userlib>:"ArmCamera.vi"("error in (no error)"=w243, "ph"=w244) -> ("error out"=w248:errorcluster, "ErrorCode"=w249:i32, "hout"=w266:u64)  [unwired: 1 in]
                        n210 = call <userlib>:"ErrorManager.vi"("ErrorIn"=w248, "ErrorCode"=w249) -> ()  [unwired: 3 in, 1 out]
                        n211 = Bundle("hout"=w266, "error out"=w248, "Description"=w268) -> (w269:T17)  [unwired: 1 in]
                        n212 = local write "Cam Variable"(w269) -> ()
                      }
                      frame #2 {
                        n213 = property on="Initialise Device" class="Ring (strict)"("DisabledEnum"=T12."Enabled" ("Disabled")) -> ()  [unwired: 2 in, 2 out]
                        "Status" <- "Camera Initialised" ("String")
                      }
                    }
                  }
                }
              }
            }
            frame #2 {
              w325 = FALSE
              n214 = property on="Finish" class="Bool"("Visible"=w325) -> ()  [unwired: 2 in, 2 out]
              n215 = property on="Status" class="Str"("Visible"=w325) -> ()  [unwired: 2 in, 2 out]
              n216 = property on="Initialise Device" class="Ring (strict)"("Visible"=w325) -> ()  [unwired: 2 in, 2 out]
            }
          }
        }
      }
    }
    frame #1 {
      n217 = local read "Motor Variable"() -> (w332:T5)
      n218 = Unbundle By Name(w332) -> ("VISA resource name"=w331:refnum<visa-resource-name>, "Axis 2"=w330:u32, "Error In"=w329:errorcluster)
      n219 = node-c288(i64 2000 ("Period")) -> (w328:T9)
      n220 = timed-loop {
        tunnel: w331 -> [w336]
        tunnel: w330 -> [w335]
        tunnel: w329 -> [w334]
        timing: w328 -> [_]
        timing-out: [_] -> w327
        stop <- w333 stop-if-true
        n221 = node-c288() -> ()  [unwired: 1 in, 1 out]
        n222 = call <userlib>:"Get Axis Motion Status.vi"("error in (no error)"=w334, "Axis (1)"=w335, "VISA resource name"=w336) -> ("Motion Done"=w333:bool)  [unwired: 2 in, 2 out]
        n223 = node-c288() -> ()  [unwired: 1 in, 1 out]
      }
      n224 = node-c288(w327) -> ()  [unwired: 1 out]
    }
    frame #2 {
      w343 = TRUE ("Visible")
      n225 = local read "Exposure in msec"() -> (w349:u32)
      n226 = local read "LCVR variable"() -> (w347:T2)
      n227 = local read "Delay in msec"() -> (w350:u32)
      n228 = property on="spectroscopy/spectropolarimetry tab" class="TabCtl (strict)"("Visible"=w343) -> ()  [unwired: 2 in, 2 out]
      n229 = property on="Close USO software" class="Bool (strict)"("Visible"=w343) -> ()  [unwired: 2 in, 2 out]
      n230 = property on="Start observation session" class="Bool (strict)"("Visible"=w343) -> ()  [unwired: 2 in, 2 out]
      n231 = property on="Cam Exp (msec)" class="DigNum (strict)"("Value"=w349) -> ()  [unwired: 2 in, 2 out]
      n232 = property on="Cam Exp (msec) sp" class="DigNum (strict)"("Value"=w349) -> ()  [unwired: 2 in, 2 out]
      n233 = property on="Cam Delay (msec) sp" class="DigNum (strict)"("Value"=w350) -> ()  [unwired: 2 in, 2 out]
      n234 = property on="Cam Delay (msec)" class="DigNum (strict)"("Value"=w350) -> ()  [unwired: 2 in, 2 out]
      n235 = Unbundle By Name(w347) -> ("LCVR Set Temperature"=w346:dbl, "Current Lcvr Temp"=w345:dbl)
      n236 = local read "Rotate in deg"() -> (w348:dbl)
      n237 = property on="Rot in deg" class="DigNum (strict)"("Value"=w348) -> ()  [unwired: 2 in, 2 out]
      n238 = property on="Rot in deg sp" class="DigNum (strict)"("Value"=w348) -> ()  [unwired: 2 in, 2 out]
      n239 = Build Array(w346, w345) -> (w344:dbl[])
      n240 = while {
        stop <- w352 stop-if-true
        # "Setup greyscale palette for intensity graph display: Color = i*(0x01 + 0x100 + 0x10000)"
        n241 = while {
          tunnel: [w1619] -> w351
          stop <- w1620 stop-if-true
          n242 = local read "Start observation session"() -> (w1621:bool)
          n243 = local read "Close USO software"() -> (w1619:bool)
          n244 = Or(x=w1619, y=w1621) -> (x .or. y?=w1620:bool)
        }
        n245 = for {
          N: 256 -> [_]
          tunnel: [w1622] -> w354 mode=indexing
          i -> [w1623]
          n246 = Multiply(x=65793, y=w1623) -> (x*y=w1622:i32)
        }
        n247 = property on="CCD Display" class="IntGraph (strict)"("Color Table"=w354) -> ()  [unwired: 2 in, 2 out]
        n248 = property on="CCD Display sp" class="IntGraph (strict)"("Color Table"=w354) -> ()  [unwired: 2 in, 2 out]
        n249 = Or(x="Close USO software", y=w351) -> (x .or. y?=w352:bool)
        n250 = case shown="False" w351 {
          frame False {
            n251 = local read "spectroscopy/spectropolarimetry tab"() -> (w356:enum32{"Spectroscopy", "Spectropolarimetry"})
            n252 = case shown="\"Spectropolarimetry\"" w356 {
              frame "Spectroscopy", Default {
                n253 = flat-sequence {
                  tunnel: [w496] -> w364
                  tunnel: [w495] -> w363
                  tunnel: [w494] -> w362
                  tunnel: [w492] -> w361
                  tunnel: w364 -> [w513]
                  tunnel: w363 -> [w508]
                  tunnel: w362 -> [w514]
                  tunnel: w361 -> [w512]
                  tunnel: [w511] -> w360
                  tunnel: [w510] -> w359
                  tunnel: [w509] -> w358
                  tunnel: [w507] -> w357
                  tunnel: w360 -> [w767]
                  tunnel: w359 -> [w770]
                  tunnel: w358 -> [w762]
                  tunnel: w357 -> [_]
                  frame #0 {
                    n254 = while {
                      stop <- w366 stop-if-true
                      n255 = while {
                        tunnel: [w373] -> w366
                        tunnel: [w376] -> w365
                        stop <- w367 stop-if-true
                        n256 = local read "Control Pannel"() -> (w374:T4)
                        n257 = Unbundle By Name(w374) -> ("Preview"=w372:bool, "Move mirror"=w371:bool, "reset motor"=w370:bool, "motor home"=w369:bool, "Restore default values"=w368:bool)
                        n258 = local read "Start Spectroscopy"() -> (w373:bool)
                        n259 = Compound Arithmetic op=OR(w372, w371, w370, w369, w368, w373) -> (w367:bool)
                        n260 = Build Array(w372, w371, w370, w369, w368) -> (w375:bool[])
                        n261 = Boolean Array To Number(Boolean array=w375) -> (number=w376:u32)
                      }
                      n262 = case shown="2" w365 {
                        frame 0, Default {
                        }
                        frame 1 {
                          w412 = u16 2 items=["nanoseconds", "microseconds", "milliseconds"] ("DelayTimeBase")
                          w397 = u32 8388608
                          # "This gives a privew image for correction or change in exposure time. NOTE exposure time set here\nwill be taken for spectroscopy unless user presses the default values button"
                          # "Preview button pressed"
                          n263 = local read "Cam Variable"() -> (w418:T6)
                          n264 = local read "Display Intensity control"() -> (w377:bool)
                          n265 = local read "Cam Delay (msec)"() -> (w390:dbl)
                          n266 = Unbundle By Name(w418) -> ("hout"=w416:u64, "ErrorOut"=w415:errorcluster, "Description"=w413:T7)
                          n267 = property on="Cam Exp (msec)" class="DigNum (strict)"() -> ("Value"=w417:dbl)  [unwired: 2 in, 2 out]
                          n268 = case shown="True" w377 {
                            frame False {
                            }
                            frame True {
                              n269 = flat-sequence {
                                frame #0 {
                                w421 = TRUE
                                n270 = property on="Slide" class="Slide (strict)"("Visible"=w421) -> ()  [unwired: 2 in, 2 out]
                                n271 = property on="accept intensity" class="Bool (strict)"("Visible"=w421) -> ()  [unwired: 2 in, 2 out]
                                }
                                frame #1 {
                                n272 = while {
                                stop <- w422 stop-if-true
                                n273 = Cluster To Array(cluster="Slide") -> (array=w426:i32[])
                                n274 = Array Max & Min(array=w426) -> (max value=w425:i32, min value=w424:i32)  [unwired: 2 out]
                                n275 = property on="CCD Display" class="IntGraph (strict)"("ZScale.Maximum"=w425, "ZScale.Minimum"=w424) -> ()  [unwired: 2 in, 2 out]
                                n276 = local read "accept intensity"() -> (w422:bool)
                                }
                                }
                                frame #2 {
                                w427 = FALSE
                                n277 = property on="Slide" class="Slide (strict)"("Visible"=w427) -> ()  [unwired: 2 in, 2 out]
                                n278 = property on="accept intensity" class="Bool (strict)"("Visible"=w427) -> ()  [unwired: 2 in, 2 out]
                                }
                              }
                            }
                          }
                          n279 = call <userlib>:"SetDelayExposureTime.vi"("ph"=w416, "Delay"=w390, "Exposure"=w417, "error in (no error)"=w415, "DelayTimeBase"=w412, "ExposureTimeBase"=w412) -> ("hout"=w405:u64, "error out"=w404:errorcluster)  [unwired: 7 in, 1 out]
                          n280 = call <userlib>:"GetRecordingState.vi"("ErrorIn"=w404, "ph"=w405) -> ("ErrorOut"=w401:errorcluster, "RecordingState"=w403:u16, "hout"=w402:u64)  [unwired: 2 in, 1 out]
                          n281 = case shown="0, Default" w403 {
                            tunnel: w402 -> [w429 w433]
                            tunnel: w401 -> [w428 w432]
                            tunnel: [w429 w431] -> w400
                            tunnel: [w428 w430] -> w399
                            frame 0, Default {
                            }
                            frame 1 {
                              w434 = u16 0 items=["Stop", "Run"] ("RecordingState")
                              n282 = call <userlib>:"SetRecordingState.vi"("ErrorIn"=w432, "RecordingState"=w434, "ph"=w433) -> ("ErrorOut"=w430:errorcluster, "hout"=w431:u64)  [unwired: 2 in, 1 out]
                            }
                          }
                          n283 = call <userlib>:"ArmCamera.vi"("error in (no error)"=w399, "ph"=w400) -> ("error out"=w394:errorcluster, "hout"=w396:u64)  [unwired: 2 out]
                          n284 = local read "Buff_no 2"() -> (w398:i16)
                          n285 = local read "Buff_no1"() -> (w411:i16)
                          n286 = call <userlib>:"ClearRAMSegment.vi"("error in (no error)"=w394, "ph"=w396) -> ("error out"=w393:errorcluster, "hout"=w395:u64)  [unwired: 1 in, 1 out]
                          n287 = call <userlib>:"AllocateBuffer.vi"("error in (no error)"=w393, "Size"=w397, "BufNr"=w398, "ph"=w395) -> ()  [unwired: 2 in, 6 out]
                          n288 = call <userlib>:"AllocateBuffer.vi"("error in (no error)"=w393, "Size"=w397, "BufNr"=w411, "ph"=w395) -> ("error out"=w409:errorcluster, "hout"=w410:u64)  [unwired: 2 in, 4 out]
                          n289 = call <userlib>:"GetRecordingState.vi"("ErrorIn"=w409, "ph"=w410) -> ("ErrorOut"=w407:errorcluster, "RecordingState"=w406:u16, "hout"=w408:u64)  [unwired: 2 in, 1 out]
                          n290 = case shown="0, Default" w406 {
                            tunnel: [w438 w441] -> w392
                            tunnel: [w437 w440] -> w391
                            tunnel: w408 -> [w436 w441]
                            tunnel: w407 -> [w435 w440]
                            frame 0, Default {
                              w439 = u16 1 items=["Stop", "Run"] ("RecordingState")
                              n291 = call <userlib>:"SetRecordingState.vi"("ErrorIn"=w435, "RecordingState"=w439, "ph"=w436) -> ("ErrorOut"=w437:errorcluster, "hout"=w438:u64)  [unwired: 2 in, 1 out]
                            }
                            frame 1 {
                            }
                          }
                          n292 = local read "Buff_no1"() -> (w386:i16)
                          n293 = call <userlib>:"ForceTrigger.vi"("ph"=w392, "error in (no error)"=w391) -> ("hout"=w387:u64, "error out"=w384:errorcluster)  [unwired: 1 in, 2 out]
                          n294 = call "grab image_2.vi"("ErrorIn"=w384, "Image number"=u32 0, "BuffNr"=w386, "ph"=w387) -> ("output image"=w378:dbl[][], "error out"=w382:errorcluster, "hout"=w383:u64)  [unwired: 4 in, 1 out]
                          n295 = local write "CCD Display"(w378) -> ()
                          n296 = Array Max & Min(array=w378) -> (max value=w381:dbl)  [unwired: 3 out]
                          n297 = call <userlib>:"CancelImages.vi"("error in (no error)"=w382, "ph"=w383) -> ("error out"=w388:errorcluster, "hout"=w389:u64)  [unwired: 1 in, 1 out]
                          n298 = Bundle("hout"=w389, "error out"=w388, "Description"=w413) -> (w414:T17)  [unwired: 1 in]
                          n299 = Greater?(x=w381, y=u16 16384) -> (0:w379:bool)
                          n300 = local write "Cam Variable"(w414) -> ()
                          n301 = case shown="True" w379 {
                            frame False {
                            }
                            frame True {
                              n302 = One Button Dialog(message="Warning CCD pixels saturated. Reduce exposure\nor reduce intensity of light              ", button name ("OK")="OK") -> ()  [unwired: 1 out]
                            }
                          }
                        }
                        frame 2 {
                          # "original value of step size given by the user while\n initiliazing is retained in motor variable"
                          # "The motor is moved by scan distance amount. NOTE If the user changes this value it will be used during spectroscopy \nrecording unless default values are being pressed"
                          # "move motor button pressed"
                          n303 = local read "Motor Variable"() -> (w447:T5)
                          n304 = Unbundle By Name(w447) -> ("VISA resource name"=w449:refnum<visa-resource-name>, "Axis 2"=w445:u32, "Error In"=w448:errorcluster)
                          n305 = local read "Rot in deg"() -> (w444:dbl)
                          n306 = call <userlib>:"Move Relative.vi"("error in (no error)"=w448, "Position (0 units)"=w444, "Axis (1)"=w445, "VISA resource name"=w449) -> ("error out"=w443:errorcluster, "VISA resource name out"=w446:refnum<visa-resource-name>)  [unwired: 2 in]
                          n307 = Bundle(cluster=w447, "VISA resource name"=w446, "Axis 2"=w445, "Error In"=w443) -> (w442:T5)  [unwired: 1 in]
                          n308 = local write "Motor Variable"(w442) -> ()
                        }
                        frame 4, 8 {
                          # "reset motor button pressed"
                          n309 = Two Button Dialog(message="Going to home position. Process cant be undone.Continue...?", 1:"No" ("F button name (\"Cancel\")"), 2:"Yes" ("T button name (\"OK\")")) -> (T button?=w453:bool)
                          n310 = case shown="True" w453 {
                            frame False {
                            }
                            frame True {
                              n311 = local read "Motor Variable"() -> (w458:T5)
                              n312 = Unbundle By Name(w458) -> ("VISA resource name"=w457:refnum<visa-resource-name>, "Axis 2"=w456:u32, "Error In"=w455:errorcluster)
                              n313 = call <userlib>:"Search For Home.vi"("Home mode"=T8."Find Positive Limit Signal", "error in (no error)"=w455, "Axis (1)"=w456, "VISA resource name"=w457) -> ()  [unwired: 3 in, 2 out]
                            }
                          }
                        }
                        frame 16 {
                          # "Restore default button pressed"
                          n314 = Two Button Dialog(message="Restore values feed during device initialization?. This process cant be undone. Continue...?", 1:"Make current as default" ("F button name (\"Cancel\")"), 2:"Restored default" ("T button name (\"OK\")")) -> (T button?=w459:bool)
                          n315 = case shown="True" w459 {
                            frame False {
                              n316 = local read "Motor Variable"() -> (w464:T5)
                              n317 = local read "Cam Exp (msec)"() -> (w467:dbl)
                              n318 = local read "Rot in deg"() -> (w466:dbl)
                              n319 = local write "Exposure in msec"(w467) -> ()
                              n320 = To Long Integer(number=w466) -> (32bit integer=w463:i32)
                              n321 = local write "Rotate in deg"(w466) -> ()
                              n322 = Bundle(cluster=w464, "Rotate in deg 2"=w463) -> (w465:T5)  [unwired: 3 in]
                              n323 = local write "Motor Variable"(w465) -> ()
                            }
                            frame True {
                              w474 = u16 2 items=["nanoseconds", "microseconds", "milliseconds"] ("DelayTimeBase")
                              n324 = local read "Cam Variable"() -> (w469:T6)
                              n325 = local read "Rotate in deg"() -> (w479:dbl)
                              n326 = local read "Exposure in msec"() -> (w476:u32)
                              n327 = local read "Delay in msec"() -> (w472:u32)
                              n328 = Unbundle By Name(w469) -> ("hout"=w478:u64, "ErrorOut"=w477:errorcluster)
                              n329 = property on="Rot in deg" class="DigNum (strict)"("Value"=w479) -> ()  [unwired: 2 in, 2 out]
                              n330 = property on="Cam Exp (msec)" class="DigNum (strict)"("Value"=w476) -> ()  [unwired: 2 in, 2 out]
                              n331 = call <userlib>:"SetDelayExposureTime.vi"("ph"=w478, "Delay"=w472, "Exposure"=w476, "error in (no error)"=w477, "DelayTimeBase"=w474) -> ("hout"=w473:u64, "error out"=w475:errorcluster)  [unwired: 8 in, 1 out]
                              n332 = call <userlib>:"ArmCamera.vi"("error in (no error)"=w475, "ph"=w473) -> ("error out"=w470:errorcluster, "hout"=w471:u64)  [unwired: 2 out]
                              n333 = Bundle(cluster=w469, "hout"=w471, "ErrorOut"=w470) -> (w468:T6)  [unwired: 1 in]
                              n334 = local write "Cam Variable"(w468) -> ()
                            }
                          }
                        }
                      }
                    }
                  }
                  frame #1 {
                    n335 = local read "Rot in deg"() -> (w482:dbl)
                    n336 = local read "Cam Variable"() -> (w498:T6)
                    n337 = Unbundle By Name(w498) -> ("hout"=w491:u64, "ErrorOut"=w490:errorcluster)
                    n338 = local read "Motor Variable"() -> (w483:T5)
                    n339 = local read "Buff_no 2"() -> (w489:i16)
                    n340 = Bundle By Name(cluster=w483, "Rotate in deg 2"=w482) -> (w481:T5)
                    n341 = call <userlib>:"AllocateBuffer.vi"("error in (no error)"=w490, "Size"=u32 8388608, "BufNr"=w489, "ph"=w491) -> ("error out"=w487:errorcluster, "BufNrOut"=w496:i16, "hout"=w488:u64)  [unwired: 2 in, 3 out]
                    n342 = local write "Motor Variable"(w481) -> ()
                    n343 = call <userlib>:"GetRecordingState.vi"("ErrorIn"=w487, "ph"=w488) -> ("ErrorOut"=w484:errorcluster, "RecordingState"=w486:u16, "hout"=w485:u64)  [unwired: 2 in, 1 out]
                    n344 = case shown="0, Default" w486 {
                      tunnel: [w503 w505] -> w495
                      tunnel: [w502 w504] -> w494
                      tunnel: w485 -> [w500 w505]
                      tunnel: w484 -> [w499 w504]
                      frame 0, Default {
                        w501 = u16 1 items=["Stop", "Run"] ("RecordingState")
                        n345 = call <userlib>:"SetRecordingState.vi"("ErrorIn"=w499, "RecordingState"=w501, "ph"=w500) -> ("ErrorOut"=w502:errorcluster, "hout"=w503:u64)  [unwired: 2 in, 1 out]
                      }
                      frame 1 {
                      }
                    }
                    n346 = call "File Dialog"("prompt"="Select folder in which data will be stored") -> ("selected path"=w480:path)  [unwired: 11 in, 3 out]
                    n347 = Path To String(path=w480) -> (string=w492:string)
                  }
                  frame #2 {
                    n348 = for {
                      N: 2 -> [_]
                      tunnel: w512 -> [w534]
                      tunnel: [w533] -> w511
                      shift-right: [w532] -> w510
                      shift-left: w514 -> [w536]
                      shift-right: [w529] -> w507
                      shift-left: w513 -> [w535]
                      shift-right: [w531] -> w509
                      shift-left: w508 -> [w530]
                      i -> [w528]
                      stop <- w524 continue-if-true
                      n349 = flat-sequence {
                        tunnel: w536 -> [w556]
                        tunnel: w535 -> [w555]
                        tunnel: w534 -> [w554]
                        tunnel: w530 -> [w550]
                        tunnel: [w542] -> w529
                        tunnel: w528 -> [w539]
                        tunnel: [w553] -> w527
                        tunnel: [w552] -> w526
                        tunnel: [w551] -> w525
                        tunnel: [w539] -> w520
                        tunnel: [w538] -> w518
                        tunnel: [w537] -> w516
                        tunnel: w527 -> [w724]
                        tunnel: w526 -> [w723]
                        tunnel: w525 -> [w722]
                        tunnel: [w718] -> w524
                        tunnel: [w724] -> w523
                        tunnel: [w723] -> w522
                        tunnel: [w722] -> w521
                        tunnel: w520 -> [w715]
                        tunnel: [w717] -> w519
                        tunnel: w518 -> [w717]
                        tunnel: [w716] -> w517
                        tunnel: w516 -> [w716]
                        tunnel: [w715] -> w515
                        tunnel: [w733] -> w531
                        tunnel: [w734] -> w532
                        tunnel: [w735] -> w533
                        tunnel: w523 -> [w735]
                        tunnel: w522 -> [w734]
                        tunnel: w521 -> [w733]
                        tunnel: w519 -> [w732]
                        tunnel: w517 -> [w731]
                        tunnel: w515 -> [w730]
                        frame #0 {
                          # "This section is to calculate the number of images stored in the cam ram. As FIFO is used after last image the image is stored from begining\nof the ram segment"
                          # "2"
                          # "These two loops must be saperate erlse camera ram wont be used and time\ntaken to cover field of view will become large"
                          n350 = local read "Scan steps"() -> (w541:dbl)
                          n351 = case shown="1" w539 {
                            tunnel: w541 -> [w557 w561]
                            tunnel: [w557 w559] -> w540
                            frame 0, Default {
                            }
                            frame 1 {
                              n352 = Divide(x=w561, y=10.0) -> (x/y=w558:dbl)
                              n353 = Round To Nearest(number=w558) -> (nearest integer value=w559:dbl)
                            }
                          }
                          n354 = for {
                            N: w540 -> [_]
                            tunnel: w550 -> [w647]
                            shift-right: [w634] -> w552
                            shift-left: w556 -> [w646]
                            shift-right: [w638] -> w547
                            shift-left: timestamp[] [] -> [w637]
                            shift-right: [w636] -> w546
                            shift-left: timestamp[] [] -> [w635]
                            tunnel: [w629] -> w538
                            tunnel: [w628] -> w537
                            i -> [w641]
                            stop <- w645 stop-if-true
                            n355 = flat-sequence {
                              tunnel: w646 -> [w651]
                              tunnel: w647 -> [w652]
                              tunnel: [w652] -> w640
                              tunnel: [w651] -> w639
                              tunnel: [w649] -> w638
                              tunnel: w637 -> [w648]
                              tunnel: [w655] -> w644
                              tunnel: [w656] -> w643
                              tunnel: w640 -> [w658]
                              tunnel: w639 -> [w657]
                              tunnel: w644 -> [w672]
                              tunnel: w643 -> [w671]
                              tunnel: [w670] -> w634
                              tunnel: [w683] -> w636
                              tunnel: w635 -> [w682]
                              tunnel: [w686] -> w633
                              tunnel: [w685] -> w632
                              tunnel: w633 -> [w691]
                              tunnel: w632 -> [w692]
                              tunnel: [w691] -> w631
                              tunnel: [w692] -> w630
                              tunnel: w631 -> [w697]
                              tunnel: w630 -> [w696]
                              tunnel: [w694] -> w627
                              tunnel: [w693] -> w626
                              tunnel: [w713] -> w628
                              tunnel: [w714] -> w629
                              tunnel: w627 -> [w714]
                              tunnel: w626 -> [w713]
                              frame #0 {
                                n356 = Get Date/Time In Seconds() -> (seconds since 1Jan1904=w650:timestamp)
                                n357 = Build Array (concatenate)(w648, w650) -> (w649:timestamp[])
                              }
                              frame #1 {
                                n358 = node-c288() -> (w654:T9)  [unwired: 1 in]
                                n359 = timed-loop {
                                shift-right: [w660] -> w655
                                shift-left: w658 -> [w663]
                                shift-right: [w661] -> w656
                                shift-left: w657 -> [w662]
                                timing: w654 -> [_]
                                timing-out: [_] -> w653
                                stop <- w659 continue-if-true
                                n360 = node-c288() -> ()  [unwired: 1 in, 1 out]
                                n361 = call <userlib>:"GetBusyStatus.vi"("error in (no error)"=w662, "ph"=w663) -> ("error out"=w661:errorcluster, "BusyState"=w659:bool, "hout"=w660:u64)  [unwired: 2 in, 1 out]
                                n362 = node-c288() -> ()  [unwired: 1 in, 1 out]
                                }
                                n363 = node-c288(w653) -> ()  [unwired: 1 out]
                              }
                              frame #2 {
                                n364 = node-c288() -> (w669:T9)  [unwired: 1 in]
                                n365 = timed-loop {
                                tunnel: w672 -> [w676]
                                shift-right: [w673] -> w670
                                shift-left: w671 -> [w674]
                                timing: w669 -> [_]
                                timing-out: [_] -> w668
                                stop <- w675 stop-if-true
                                n366 = node-c288() -> ()  [unwired: 1 in, 1 out]
                                n367 = call <userlib>:"ForceTrigger.vi"("ph"=w676, "error in (no error)"=w674) -> ("Triggered"=w675:bool, "error out"=w673:errorcluster)  [unwired: 1 in, 2 out]
                                n368 = node-c288() -> ()  [unwired: 1 in, 1 out]
                                }
                                n369 = node-c288(w668) -> ()  [unwired: 1 out]
                              }
                              frame #3 {
                                n370 = local read "Exposure in msec"() -> (w681:u32)
                                n371 = Wait (ms)(milliseconds to wait=w681) -> ()  [unwired: 1 out]
                              }
                              frame #4 {
                                n372 = Get Date/Time In Seconds() -> (seconds since 1Jan1904=w684:timestamp)
                                n373 = Build Array (concatenate)(w682, w684) -> (w683:timestamp[])
                              }
                              frame #5 {
                                n374 = local read "Motor Variable"() -> (w690:T5)
                                n375 = Unbundle By Name(w690) -> ("VISA resource name"=w689:refnum<visa-resource-name>, "Axis 2"=w685:u32, "Rotate in deg 2"=w688:dbl, "Error In"=w687:errorcluster)
                                n376 = call <userlib>:"Move Relative.vi"("error in (no error)"=w687, "Position (0 units)"=w688, "Axis (1)"=w685, "VISA resource name"=w689) -> ("VISA resource name out"=w686:refnum<visa-resource-name>)  [unwired: 2 in, 1 out]
                              }
                              frame #6 {
                              }
                              frame #7 {
                                n377 = node-c288() -> (w699:T9)  [unwired: 1 in]
                                n378 = timed-loop {
                                tunnel: w697 -> [w707]
                                tunnel: w696 -> [w700]
                                shift-right: [w705] -> _
                                shift-left: 1000.0 ("Position (units)") -> [w706]
                                timing: w699 -> [_]
                                timing-out: [_] -> w698
                                tunnel: [w701] -> w694
                                tunnel: [w700] -> w693
                                stop <- w702 stop-if-true
                                n379 = node-c288() -> ()  [unwired: 1 in, 1 out]
                                n380 = call <userlib>:"Read Actual Position.vi"("Axis (1)"=w700, "VISA resource name"=w707) -> ("Position (units)"=w705:dbl, "VISA resource name out"=w701:refnum<visa-resource-name>)  [unwired: 3 in, 1 out]
                                n381 = Subtract(x=w706, y=w705) -> (x-y=w704:dbl)
                                n382 = Equal?(x=w704, y=0.0) -> (x = y?=w702:bool)
                                n383 = node-c288() -> ()  [unwired: 1 in, 1 out]
                                }
                                n384 = node-c288(w698) -> ()  [unwired: 1 out]
                              }
                              frame #8 {
                                # "I am forced to use this delay\nas my motor has very bad settling \ntime"
                                n385 = Wait (ms)(milliseconds to wait=u32 5000) -> ()  [unwired: 1 out]
                              }
                            }
                            n386 = Increment(x=w641) -> (x+1=w642:i32)
                            n387 = local write "Steps performed"(w642) -> ()
                            n388 = local read "Stop Spectroscopy"() -> (w645:bool)
                          }
                          n389 = property on="Steps performed" class="Slide (strict)"("Scale.Maximum"=w540) -> ()  [unwired: 2 in, 2 out]
                          n390 = local write "End time Array"(w546) -> ()
                          n391 = local write "Start time Array"(w547) -> ()
                          n392 = Initialize Array(0.0 ("element"), 4 ("dimension size")) -> (w543:dbl[])
                          n393 = for {
                            N: w540 -> [w590]
                            tunnel: w550 -> [w621]
                            tunnel: w555 -> [w566]
                            tunnel: w554 -> [w619]
                            shift-right: [w615] -> w553
                            shift-left: w556 -> [w620]
                            tunnel: [w611] -> w551
                            tunnel: w543 -> [w587]
                            tunnel: w543 -> [w578]
                            tunnel: [w566] -> w542
                            tunnel: w539 -> [w565]
                            i -> [w568]
                            stop <- w616 stop-if-true
                            w607 = T18 16 items=["<invalid type>"=0, "BYTE_IMG  (U8)"=8, "SHORT_IMG  (I16)"=16, "USHORT_IMG  (U16)"=20, "LONG_IMG  (I32)"=32, "ULONG_IMG  (U32)"=40, "FLOAT_IMG  (SGL)"=-32, "DOUBLE_IMG  (DBL)"=-64] ("image data type")
                            n394 = case shown="0, Default" w565 {
                              tunnel: ["data_" "flat_"] -> w562
                              frame 0, Default {
                              }
                              frame 1 {
                              }
                            }
                            n395 = Format Into String(format string="%04d", w568) -> (resulting string=w563:string)  [unwired: 2 in, 1 out]
                            n396 = call "grab image_2.vi"("ErrorIn"=w620, "Image number"=u32 0, "BuffNr"=w566, "ph"=w621) -> ("output image"=w602:dbl[][], "error out"=w615:errorcluster, "hout"=w611:u64)  [unwired: 4 in, 1 out]
                            n397 = local write "CCD Display"(w602) -> ()
                            n398 = Concatenate Strings(w619, "\\" ("string"), w562, w563, ".fits" ("string")) -> (w617:string)
                            n399 = String To Path(string=w617) -> (path=w614:path)
                            n400 = local read "Exposure in msec"() -> (w589:u32)
                            n401 = call "gfitsio-open-create-replace-file.vi"("function (open)"=T13."open or create", "file path (dialog if empty)"=w614) -> ("error out"=w608:errorcluster, "new file path"=w601:path, "gfits refnum"=w609:T19)  [unwired: 7 in]
                            n402 = Initialize Array(i16 2048 ("element"), 2 ("dimension size")) -> (w605:i16[])
                            n403 = call "gfitsio-resize-image.vi"("image data type"=w607, "naxes"=w605, "error in (no error)"=w608, "gfits refnum"=w609) -> ("error out"=w598:errorcluster, "dup gfits refnum"=w600:T19)  [unwired: 6 in]
                            n404 = local read "End time Array"() -> (w593:timestamp[])
                            n405 = local write "Data is stored in the folder........."(w601) -> ()
                            n406 = case shown="0" w568 {
                              tunnel: [TRUE FALSE] -> w569
                              frame 0 {
                              }
                              frame 1, Default {
                              }
                            }
                            n407 = local read "Start time Array"() -> (w596:timestamp[])
                            n408 = Increment(x=w568) -> (x+1=w588:i32)
                            n409 = Index Array(array=w593, index=0) -> (element=w591:timestamp)
                            n410 = Index Array(array=w596, index=0) -> (element=w594:timestamp)
                            n411 = local read "Stop Spectroscopy"() -> (w616:bool)
                            n412 = Index Array(array=w578, index=0) -> (element=w573:dbl)
                            n413 = Index Array(array=w578, index=1) -> (element=w572:dbl)
                            n414 = Index Array(array=w578, index=2) -> (element=w571:dbl)
                            n415 = Index Array(array=w578, index=3) -> (element=w570:dbl)
                            n416 = Index Array(array=w587, index=2) -> (element=w580:dbl)
                            n417 = Index Array(array=w587, index=1) -> (element=w581:dbl)
                            n418 = Index Array(array=w587, index=3) -> (element=w579:dbl)
                            n419 = Index Array(array=w587, index=0) -> (element=w582:dbl)
                            n420 = call "fits_header.vi"("gfits refnum"=w600, "error in (no error)"=w598, "start time"=w594, "total scans"=w590, "end time"=w591, "Exposure"=w589, "lcvr1_2"=w581, "lcvr2_4"=w570, "lcvr1_4"=w579, "lcvr2_2"=w572, "lcvr1_1"=w582, "lcvr1_3"=w580, "lcvr2_1"=w573, "lcvr2_3"=w571, "Curr Scan"=w588, "Teliscope parameters"=w569) -> ("dup gfits refnum"=w599:T19, "error out"=w597:errorcluster)  [unwired: 10 in]
                            n421 = call "gfitsio-write-image-subset-i16-2d.vi"("error in (no error)"=w597, "data"=w602, "gfits refnum"=w599) -> ("error out"=w603:errorcluster, "dup gfits refnum"=w612:T19)  [unwired: 7 in]
                            n422 = call "gfitsio-close-file.vi"("error in (no error)"=w603, "gfits refnum"=w612) -> ()  [unwired: 8 in, 2 out]
                          }
                        }
                        frame #1 {
                          n423 = case shown="0, Default" w715 {
                            tunnel: [w726 FALSE ("T button?")] -> w719
                            frame 0, Default {
                              n424 = Two Button Dialog(message="Going for flat field. If yes move\nteliscope to quiet sun and start \nmoving it before clicking on \"yes\"", 1:"No" ("F button name (\"Cancel\")"), 2:"Yes" ("T button name (\"OK\")")) -> (T button?=w726:bool)
                            }
                            frame 1 {
                            }
                          }
                          n425 = local read "Stop Spectroscopy"() -> (w721:bool)
                          n426 = Not(x=w721) -> (.not. x?=w720:bool)
                          n427 = And(x=w720, y=w719) -> (x .and. y?=w718:bool)
                        }
                        frame #2 {
                          n428 = case shown="0, Default" w730 {
                            tunnel: w732 -> [w751 w761]
                            tunnel: w731 -> [w750 w760]
                            frame 0, Default {
                              # "This gives mid point"
                              n429 = local read "Motor Variable"() -> (w749:T5)
                              n430 = Unbundle By Name(w749) -> ("Rotate in deg 2"=w741:dbl)
                              n431 = local read "Scan steps"() -> (w744:dbl)
                              n432 = local read "initial absolute position"() -> (w745:dbl)
                              n433 = Multiply(x=w741, y=w744) -> (x*y=w748:dbl)
                              n434 = Divide(x=w744, y=10.0) -> (x/y=w742:dbl)
                              n435 = Multiply(x=w742, y=w741) -> (x*y=w740:dbl)
                              n436 = Divide(x=w748, y=2.0) -> (x/y=w746:dbl)
                              n437 = Add(x=w746, y=w745) -> (x+y=w738:dbl)
                              n438 = Divide(x=w740, y=2.0) -> (x/y=w737:dbl)
                              n439 = Subtract(x=w738, y=w737) -> (x-y=w736:dbl)
                              n440 = call <userlib>:"Move Absolute.vi"("Position (0 units)"=w736, "Axis (1)"=w750, "VISA resource name"=w751) -> ()  [unwired: 3 in, 2 out]
                            }
                            frame 1 {
                              n441 = local read "Motor Variable"() -> (w759:T5)
                              n442 = Unbundle By Name(w759) -> ("Rotate in deg 2"=w758:dbl)
                              n443 = local read "Scan steps"() -> (w757:dbl)
                              n444 = local read "initial absolute position"() -> (w753:dbl)
                              n445 = Multiply(x=w758, y=w757) -> (x*y=w756:dbl)
                              n446 = Divide(x=w756, y=2.0) -> (x/y=w754:dbl)
                              n447 = Add(x=w754, y=w753) -> (x+y=w752:dbl)
                              n448 = call <userlib>:"Move Absolute.vi"("Position (0 units)"=w752, "Axis (1)"=w760, "VISA resource name"=w761) -> ()  [unwired: 3 in, 2 out]
                            }
                          }
                        }
                      }
                    }
                  }
                  frame #3 {
                    n449 = Merge Errors(w770, w767) -> (w769:errorcluster)
                    n450 = call <userlib>:"CancelImages.vi"("error in (no error)"=w767, "ph"=w762) -> ("error out"=w764:errorcluster, "hout"=w765:u64)  [unwired: 1 in, 1 out]
                    n451 = call <vilib>:"Simple Error Handler.vi"("error in (no error)"=w769) -> ()  [unwired: 4 in, 5 out]
                    n452 = local read "Cam Variable"() -> (w766:T6)
                    n453 = local read "Stop Spectroscopy"() -> (w768:bool)
                    n454 = Bundle(cluster=w766, "hout"=w765, "ErrorOut"=w764) -> (w763:T6)  [unwired: 1 in]
                    n455 = local write "Cam Variable"(w763) -> ()
                    n456 = case shown="True" w768 {
                      frame False {
                        n457 = flat-sequence {
                          frame #0 {
                            n458 = Two Button Dialog(message="Spectroscopy completed successfully!!.    Reset Motor?", 1:"No" ("button name (\"OK\")"), 2:"Yes" ("T button name (\"OK\")")) -> (T button?=w771:bool)
                            n459 = case shown="True" w771 {
                              frame False {
                              }
                              frame True {
                                n460 = local read "Motor Variable"() -> (w779:T5)
                                n461 = Unbundle By Name(w779) -> ("VISA resource name"=w778:refnum<visa-resource-name>, "Axis 2"=w777:u32, "Error In"=w776:errorcluster)
                                n462 = local read "initial absolute position"() -> (w775:dbl)
                                n463 = call <userlib>:"Move Absolute.vi"("error in (no error)"=w776, "Position (0 units)"=w775, "Axis (1)"=w777, "VISA resource name"=w778) -> ()  [unwired: 2 in, 2 out]
                              }
                            }
                          }
                        }
                      }
                      frame True {
                        n464 = local write "Stop Spectroscopy"(FALSE ("Stop Spectroscopy")) -> ()
                        n465 = Two Button Dialog(message="Spectroscopy Stopped by user. Reset motor?", 1:"No" ("F button name (\"Cancel\")"), 2:"Yes" ("T button name (\"OK\")")) -> (T button?=w781:bool)
                        n466 = case shown="False" w781 {
                          frame False {
                          }
                          frame True {
                            n467 = local read "Motor Variable"() -> (w789:T5)
                            n468 = Unbundle By Name(w789) -> ("VISA resource name"=w788:refnum<visa-resource-name>, "Axis 2"=w787:u32, "Error In"=w786:errorcluster)
                            n469 = local read "initial absolute position"() -> (w785:dbl)
                            n470 = call <userlib>:"Move Absolute.vi"("error in (no error)"=w786, "Position (0 units)"=w785, "Axis (1)"=w787, "VISA resource name"=w788) -> ()  [unwired: 2 in, 2 out]
                          }
                        }
                      }
                    }
                  }
                }
              }
              frame "Spectropolarimetry" {
                n471 = local read "LCVR variable"() -> (w796:T2)
                n472 = Unbundle By Name(w796) -> ("Open USB I/O Stuff"=w797:T14, "Current Lcvr Temp"=w798:dbl)  [unwired: 1 out]
                n473 = while {
                  shift-right: [w815] -> w795
                  shift-left: w797 -> [w815]
                  shift-right: [w820] -> w793
                  shift-left: w798 -> [w814]
                  i -> [w808]
                  stop <- w810 stop-if-true
                  n474 = call "read temp.vi"("USB Open Device Cluster"=w815) -> ("Temp"=w820:dbl)
                  n475 = local read "Stop Spectroscopy sp"() -> (w811:bool)
                  n476 = Equal?(x=w808, y=10) -> (x = y?=w806:bool)
                  n477 = local read "Close USO software"() -> (w812:bool)
                  n478 = local read "LCVR Temperature in deg C\n      Set         Current"() -> (w819:dbl[])
                  n479 = Compound Arithmetic op=OR(w812, w811, w806) -> (w810:bool)
                  n480 = local read "LCVR Set Temperature"() -> (w816:dbl)
                  n481 = Index Array(array=w819, index=0) -> (element=w809:dbl)
                  n482 = Not Equal?(x=w809, y=w816) -> (x != y?=w817:bool)
                  n483 = Build Array(w809, w814) -> (w813:dbl[])
                  n484 = case shown="True" w817 {
                    tunnel: w809 -> [_ w821]
                    tunnel: w815 -> [_ w822]
                    frame False {
                    }
                    frame True {
                      n485 = call "Set temp.vi"("Temp"=w821, "USB Open Device Cluster"=w822) -> ()  [unwired: 1 in]
                      n486 = local write "LCVR Set Temperature"(w821) -> ()
                    }
                  }
                  n487 = local write "LCVR Temperature in deg C\n      Set         Current"(w813) -> ()
                }
                n488 = flat-sequence {
                  tunnel: [w958] -> w805
                  tunnel: [w957] -> w804
                  tunnel: [w956] -> w803
                  tunnel: [w954] -> w802
                  tunnel: [w945] -> w791
                  tunnel: w805 -> [w975]
                  tunnel: w804 -> [w976]
                  tunnel: w803 -> [w974]
                  tunnel: w802 -> [w972]
                  tunnel: [w971] -> w801
                  tunnel: [w977] -> w800
                  tunnel: [w973] -> w799
                  tunnel: [w970] -> w792
                  tunnel: w791 -> [w970]
                  tunnel: [w969] -> w790
                  tunnel: w801 -> [w1582]
                  tunnel: w800 -> [w1585]
                  tunnel: w799 -> [w1581]
                  tunnel: w792 -> [w1580]
                  tunnel: w790 -> [w1579]
                  frame #0 {
                    n489 = while {
                      stop <- w823 stop-if-true
                      n490 = while {
                        tunnel: [w834] -> w824
                        tunnel: [w825] -> w823
                        stop <- w826 stop-if-true
                        n491 = local read "Control Pannel sp"() -> (w832:T4)
                        n492 = Unbundle By Name(w832) -> ("Preview"=w831:bool, "Move mirror"=w830:bool, "reset motor"=w829:bool, "motor home"=w828:bool, "Restore default values"=w827:bool)
                        n493 = local read "Start Spectroscopy sp"() -> (w825:bool)
                        n494 = Compound Arithmetic op=OR(w831, w830, w829, w828, w827, w825) -> (w826:bool)
                        n495 = Build Array(w831, w830, w829, w828, w827) -> (w833:bool[])
                        n496 = Boolean Array To Number(Boolean array=w833) -> (number=w834:u32)
                      }
                      n497 = case shown="16" w824 {
                        frame 0, Default {
                        }
                        frame 1 {
                          w871 = u16 2 items=["nanoseconds", "microseconds", "milliseconds"] ("DelayTimeBase")
                          w856 = u32 8388608
                          # "This gives a privew image for correction or change in exposure time. NOTE exposure time set here\nwill be taken for spectroscopy unless user presses the default values button"
                          # "Preview button pressed"
                          n498 = local read "Cam Variable"() -> (w876:T6)
                          n499 = local read "Cam Delay (msec) sp"() -> (w849:dbl)
                          n500 = property on="Cam Exp (msec) sp" class="DigNum (strict)"() -> ("Value"=w835:dbl)  [unwired: 2 in, 2 out]
                          n501 = Unbundle By Name(w876) -> ("hout"=w875:u64, "ErrorOut"=w874:errorcluster, "Description"=w872:T7)
                          n502 = local read "Display Intensity control sp"() -> (w836:bool)
                          n503 = call <userlib>:"SetDelayExposureTime.vi"("ph"=w875, "Delay"=w849, "Exposure"=w835, "error in (no error)"=w874, "DelayTimeBase"=w871, "ExposureTimeBase"=w871) -> ("hout"=w864:u64, "error out"=w863:errorcluster)  [unwired: 7 in, 1 out]
                          n504 = case shown="True" w836 {
                            frame False {
                            }
                            frame True {
                              n505 = flat-sequence {
                                frame #0 {
                                w879 = TRUE
                                n506 = property on="Slide sp" class="Slide (strict)"("Visible"=w879) -> ()  [unwired: 2 in, 2 out]
                                n507 = property on="accept intensity sp" class="Bool (strict)"("Visible"=w879) -> ()  [unwired: 2 in, 2 out]
                                }
                                frame #1 {
                                n508 = while {
                                stop <- w883 stop-if-true
                                n509 = Cluster To Array(cluster="Slide sp") -> (array=w884:i32[])
                                n510 = Array Max & Min(array=w884) -> (max value=w881:i32, min value=w880:i32)  [unwired: 2 out]
                                n511 = property on="CCD Display sp" class="IntGraph (strict)"("ZScale.Maximum"=w881, "ZScale.Minimum"=w880) -> ()  [unwired: 2 in, 2 out]
                                n512 = local read "accept intensity sp"() -> (w883:bool)
                                }
                                }
                                frame #2 {
                                w885 = FALSE
                                n513 = property on="Slide sp" class="Slide (strict)"("Visible"=w885) -> ()  [unwired: 2 in, 2 out]
                                n514 = property on="accept intensity sp" class="Bool (strict)"("Visible"=w885) -> ()  [unwired: 2 in, 2 out]
                                }
                              }
                            }
                          }
                          n515 = call <userlib>:"GetRecordingState.vi"("ErrorIn"=w863, "ph"=w864) -> ("ErrorOut"=w860:errorcluster, "RecordingState"=w862:u16, "hout"=w861:u64)  [unwired: 2 in, 1 out]
                          n516 = case shown="0, Default" w862 {
                            tunnel: w861 -> [w887 w891]
                            tunnel: w860 -> [w886 w890]
                            tunnel: [w887 w889] -> w859
                            tunnel: [w886 w888] -> w858
                            frame 0, Default {
                            }
                            frame 1 {
                              w892 = u16 0 items=["Stop", "Run"] ("RecordingState")
                              n517 = call <userlib>:"SetRecordingState.vi"("ErrorIn"=w890, "RecordingState"=w892, "ph"=w891) -> ("ErrorOut"=w888:errorcluster, "hout"=w889:u64)  [unwired: 2 in, 1 out]
                            }
                          }
                          n518 = call <userlib>:"ArmCamera.vi"("error in (no error)"=w858, "ph"=w859) -> ("error out"=w853:errorcluster, "hout"=w855:u64)  [unwired: 2 out]
                          n519 = local read "Buff_no 2"() -> (w857:i16)
                          n520 = local read "Buff_no1"() -> (w870:i16)
                          n521 = call <userlib>:"ClearRAMSegment.vi"("error in (no error)"=w853, "ph"=w855) -> ("error out"=w852:errorcluster, "hout"=w854:u64)  [unwired: 1 in, 1 out]
                          n522 = call <userlib>:"AllocateBuffer.vi"("error in (no error)"=w852, "Size"=w856, "BufNr"=w857, "ph"=w854) -> ()  [unwired: 2 in, 6 out]
                          n523 = call <userlib>:"AllocateBuffer.vi"("error in (no error)"=w852, "Size"=w856, "BufNr"=w870, "ph"=w854) -> ("error out"=w868:errorcluster, "hout"=w869:u64)  [unwired: 2 in, 4 out]
                          n524 = call <userlib>:"GetRecordingState.vi"("ErrorIn"=w868, "ph"=w869) -> ("ErrorOut"=w866:errorcluster, "RecordingState"=w865:u16, "hout"=w867:u64)  [unwired: 2 in, 1 out]
                          n525 = case shown="0, Default" w865 {
                            tunnel: [w896 w899] -> w851
                            tunnel: [w895 w898] -> w850
                            tunnel: w867 -> [w894 w899]
                            tunnel: w866 -> [w893 w898]
                            frame 0, Default {
                              w897 = u16 1 items=["Stop", "Run"] ("RecordingState")
                              n526 = call <userlib>:"SetRecordingState.vi"("ErrorIn"=w893, "RecordingState"=w897, "ph"=w894) -> ("ErrorOut"=w895:errorcluster, "hout"=w896:u64)  [unwired: 2 in, 1 out]
                            }
                            frame 1 {
                            }
                          }
                          n527 = local read "Buff_no1"() -> (w845:i16)
                          n528 = call <userlib>:"ForceTrigger.vi"("ph"=w851, "error in (no error)"=w850) -> ("hout"=w846:u64, "error out"=w843:errorcluster)  [unwired: 1 in, 2 out]
                          n529 = call "grab image_2.vi"("ErrorIn"=w843, "Image number"=u32 0, "BuffNr"=w845, "ph"=w846) -> ("output image"=w837:dbl[][], "error out"=w841:errorcluster, "hout"=w842:u64)  [unwired: 4 in, 1 out]
                          n530 = Array Max & Min(array=w837) -> (max value=w840:dbl)  [unwired: 3 out]
                          n531 = local write "CCD Display sp"(w837) -> ()
                          n532 = call <userlib>:"CancelImages.vi"("error in (no error)"=w841, "ph"=w842) -> ("error out"=w847:errorcluster, "hout"=w848:u64)  [unwired: 1 in, 1 out]
                          n533 = Bundle("hout"=w848, "error out"=w847, "Description"=w872) -> (w873:T17)  [unwired: 1 in]
                          n534 = Greater?(x=w840, y=u16 16384) -> (0:w838:bool)
                          n535 = local write "Cam Variable"(w873) -> ()
                          n536 = case shown="False" w838 {
                            frame False {
                            }
                            frame True {
                              n537 = One Button Dialog(message="Warning CCD pixels saturated. Reduce exposure\nor reduce intensity of light              ", button name ("OK")="OK") -> ()  [unwired: 1 out]
                            }
                          }
                        }
                        frame 2 {
                          # "original value of step size given by the user while\n initiliazing is retained in motor variable"
                          # "The motor is moved by scan distance amount. NOTE If the user changes this value it will be used during spectroscopy \nrecording unless default values are being pressed"
                          # "move motor button pressed"
                          n538 = local read "Motor Variable"() -> (w904:T5)
                          n539 = local read "Rot in deg sp"() -> (w901:dbl)
                          n540 = Unbundle By Name(w904) -> ("VISA resource name"=w903:refnum<visa-resource-name>, "Axis 2"=w902:u32, "Error In"=w900:errorcluster)
                          n541 = call <userlib>:"Move Relative.vi"("error in (no error)"=w900, "Position (0 units)"=w901, "Axis (1)"=w902, "VISA resource name"=w903) -> ()  [unwired: 2 in, 2 out]
                        }
                        frame 4, 8 {
                          # "motor has backlash. so if current position is not 0\nwe itterate to come to zero"
                          # "reset motor button pressed"
                          n542 = Two Button Dialog(message="Going to home position. Process cant be undone.Continue...?", 1:"No" ("F button name (\"Cancel\")"), 2:"Yes" ("T button name (\"OK\")")) -> (T button?=w908:bool)
                          n543 = case shown="True" w908 {
                            frame False {
                            }
                            frame True {
                              n544 = local read "Motor Variable"() -> (w913:T5)
                              n545 = Unbundle By Name(w913) -> ("VISA resource name"=w912:refnum<visa-resource-name>, "Axis 2"=w911:u32, "Error In"=w910:errorcluster)
                              n546 = call <userlib>:"Search For Home.vi"("Home mode"=T8."Find Positive Limit Signal", "error in (no error)"=w910, "Axis (1)"=w911, "VISA resource name"=w912) -> ()  [unwired: 3 in, 2 out]
                            }
                          }
                        }
                        frame 16 {
                          # "Restore default button pressed"
                          n547 = Two Button Dialog(message="Restore values feed during device initialization?. This process cant be undone. Continue...?", 1:"Make current as default" ("F button name (\"Cancel\")"), 2:"Restored default" ("T button name (\"OK\")")) -> (T button?=w914:bool)
                          n548 = case shown="False" w914 {
                            frame False {
                              n549 = local read "Cam Exp (msec) sp"() -> (w922:dbl)
                              n550 = local read "Rot in deg sp"() -> (w921:dbl)
                              n551 = local write "Exposure in msec"(w922) -> ()
                              n552 = local read "Motor Variable"() -> (w920:T5)
                              n553 = To Long Integer(number=w921) -> (32bit integer=w919:i32)
                              n554 = local write "Rotate in deg"(w921) -> ()
                              n555 = Bundle(cluster=w920, "Rotate in deg 2"=w919) -> (w918:T5)  [unwired: 3 in]
                              n556 = local write "Motor Variable"(w918) -> ()
                            }
                            frame True {
                              w930 = u16 2 items=["nanoseconds", "microseconds", "milliseconds"] ("DelayTimeBase")
                              n557 = local read "Cam Variable"() -> (w925:T6)
                              n558 = local read "Rotate in deg"() -> (w923:dbl)
                              n559 = local read "Exposure in msec"() -> (w932:u32)
                              n560 = local read "Delay in msec"() -> (w928:u32)
                              n561 = Unbundle By Name(w925) -> ("hout"=w934:u64, "ErrorOut"=w933:errorcluster)
                              n562 = property on="Rot in deg sp" class="DigNum (strict)"("Value"=w923) -> ()  [unwired: 2 in, 2 out]
                              n563 = call <userlib>:"SetDelayExposureTime.vi"("ph"=w934, "Delay"=w928, "Exposure"=w932, "error in (no error)"=w933, "DelayTimeBase"=w930) -> ("hout"=w929:u64, "error out"=w931:errorcluster)  [unwired: 8 in, 1 out]
                              n564 = call <userlib>:"ArmCamera.vi"("error in (no error)"=w931, "ph"=w929) -> ("error out"=w926:errorcluster, "hout"=w927:u64)  [unwired: 2 out]
                              n565 = Bundle(cluster=w925, "hout"=w927, "ErrorOut"=w926) -> (w924:T6)  [unwired: 1 in]
                              n566 = local write "Cam Variable"(w924) -> ()
                            }
                          }
                        }
                      }
                    }
                  }
                  frame #1 {
                    n567 = local read "LCVR variable"() -> (w942:T2)
                    n568 = local read "Rot in deg sp"() -> (w936:dbl)
                    n569 = local read "Motor Variable"() -> (w937:T5)
                    n570 = Unbundle By Name(w942) -> ("LCVR Set Temperature"=w941:dbl, "Current Lcvr Temp"=w940:dbl)
                    n571 = Bundle By Name(cluster=w937, "Rotate in deg 2"=w936) -> (w935:T5)
                    n572 = call "= to within Tolerance"("Operand 2"=w940, "Operand 1"=w941) -> ("Result"=w939:dynamicdata)  [unwired: 8 in, 1 out]
                    n573 = call "Convert from Dynamic Data"("Dynamic Data Type"=w939) -> ("Scalar"=w938:bool)  [unwired: 3 in]
                    n574 = case shown="False" w938 {
                      frame False {
                        n575 = One Button Dialog(message="Warning the lcvr temp \nis not equal to the set temp", button name ("OK")="OK") -> ()  [unwired: 1 out]
                      }
                      frame True {
                      }
                    }
                    n576 = local write "Motor Variable"(w935) -> ()
                  }
                  frame #2 {
                    n577 = local read "Cam Variable"() -> (w960:T6)
                    n578 = local read "Buff_no 2"() -> (w951:i16)
                    n579 = Unbundle By Name(w960) -> ("hout"=w953:u64, "ErrorOut"=w952:errorcluster)
                    n580 = call <userlib>:"AllocateBuffer.vi"("error in (no error)"=w952, "Size"=u32 8388608, "BufNr"=w951, "ph"=w953) -> ("error out"=w949:errorcluster, "BufNrOut"=w958:i16, "hout"=w950:u64)  [unwired: 2 in, 3 out]
                    n581 = call <userlib>:"GetRecordingState.vi"("ErrorIn"=w949, "ph"=w950) -> ("ErrorOut"=w946:errorcluster, "RecordingState"=w948:u16, "hout"=w947:u64)  [unwired: 2 in, 1 out]
                    n582 = case shown="0, Default" w948 {
                      tunnel: [w965 w967] -> w957
                      tunnel: [w964 w966] -> w956
                      tunnel: w947 -> [w962 w967]
                      tunnel: w946 -> [w961 w966]
                      frame 0, Default {
                        w963 = u16 1 items=["Stop", "Run"] ("RecordingState")
                        n583 = call <userlib>:"SetRecordingState.vi"("ErrorIn"=w961, "RecordingState"=w963, "ph"=w962) -> ("ErrorOut"=w964:errorcluster, "hout"=w965:u64)  [unwired: 2 in, 1 out]
                      }
                      frame 1 {
                      }
                    }
                    n584 = call "File Dialog2"("prompt"="Select folder in which data will be stored") -> ("selected path"=w945:path)  [unwired: 11 in, 3 out]
                    n585 = Path To String(path=w945) -> (string=w954:string)
                  }
                  frame #3 {
                    n586 = for {
                      N: 2 -> [_]
                      tunnel: w972 -> [w992]
                      tunnel: [w991] -> w971
                      shift-right: [w993] -> w973
                      shift-left: w976 -> [w996]
                      shift-right: [w990] -> w969
                      shift-left: w975 -> [w995]
                      shift-right: [w997] -> w977
                      shift-left: w974 -> [w994]
                      i -> [w989]
                      stop <- w985 continue-if-true
                      n587 = flat-sequence {
                        tunnel: w996 -> [w1015]
                        tunnel: w995 -> [w1014]
                        tunnel: w994 -> [w1013]
                        tunnel: [w1012] -> w993
                        tunnel: w992 -> [w1011]
                        tunnel: [w1005] -> w990
                        tunnel: w989 -> [w1001]
                        tunnel: [w1017] -> w988
                        tunnel: [w1010] -> w987
                        tunnel: [w1001] -> w986
                        tunnel: [w1000] -> w981
                        tunnel: [w999] -> w979
                        tunnel: w988 -> [w1542]
                        tunnel: w987 -> [w1541]
                        tunnel: w986 -> [w1534]
                        tunnel: [w1537] -> w985
                        tunnel: [w1542] -> w984
                        tunnel: [w1541] -> w983
                        tunnel: [w1536] -> w982
                        tunnel: w981 -> [w1536]
                        tunnel: [w1535] -> w980
                        tunnel: w979 -> [w1535]
                        tunnel: [w1534] -> w978
                        tunnel: [w1551] -> w991
                        tunnel: [w1552] -> w997
                        tunnel: w984 -> [w1552]
                        tunnel: w983 -> [w1551]
                        tunnel: w982 -> [w1550]
                        tunnel: w980 -> [w1549]
                        tunnel: w978 -> [w1548]
                        frame #0 {
                          # "This section is to calculate the number of images stored in the cam ram. As FIFO is used after last image the image is stored from begining\nof the ram segment"
                          n588 = local read "Image averaging"() -> (w1016:enum32{"Per scan", "Per Polarisation"})
                          n589 = local read "Averaging \nNum"() -> (w1004:dbl)
                          n590 = local read "Scan steps sp"() -> (w1003:dbl)
                          n591 = case shown="1" w1001 {
                            tunnel: [w1018 1.0 ("Averaging \nNum")] -> w1002
                            tunnel: w1004 -> [w1018 _]
                            frame 0, Default {
                            }
                            frame 1 {
                            }
                          }
                          n592 = case shown="1" w1001 {
                            tunnel: [w1020 w1021] -> w998
                            tunnel: w1003 -> [w1020 w1024]
                            frame 0, Default {
                            }
                            frame 1 {
                              n593 = Divide(x=w1024, y=10.0) -> (x/y=w1022:dbl)
                              n594 = Round To Nearest(number=w1022) -> (nearest integer value=w1021:dbl)
                            }
                          }
                          n595 = property on="Steps performed sp" class="Slide (strict)"("Scale.Maximum"=w998) -> ()  [unwired: 2 in, 2 out]
                          n596 = case shown="\"Per Polarisation\"" w1016 {
                            tunnel: w1015 -> [w1037 w1203]
                            tunnel: w1014 -> [w1036 w1202]
                            tunnel: w1013 -> [w1035 w1201]
                            tunnel: [w1034 w1200] -> w1012
                            tunnel: w1002 -> [w1032 w1199]
                            tunnel: w998 -> [w1033 w1198]
                            tunnel: w1011 -> [w1031 w1197]
                            tunnel: [w1030 w1196] -> w1010
                            tunnel: [w1026 w1192] -> w1005
                            tunnel: w1001 -> [w1025 w1191]
                            frame "Per scan", Default {
                              n597 = local read "LCVR variable"() -> (w1029:T2)
                              n598 = Unbundle By Name(w1029) -> ("volt set of lcvr 1"=w1028:dbl[], "volt set of lcvr 2"=w1027:dbl[])
                              n599 = for {
                                N: w1033 -> [w1062]
                                tunnel: w1036 -> [w1111]
                                tunnel: w1035 -> [w1110]
                                tunnel: w1032 -> [w1060]
                                shift-right: [w1109] -> w1034
                                shift-left: w1037 -> [w1112]
                                tunnel: w1032 -> [w1104]
                                tunnel: w1031 -> [w1102]
                                tunnel: [w1086] -> w1030
                                tunnel: w1028 -> [w1046]
                                tunnel: w1027 -> [w1045]
                                tunnel: [w1042] -> w1026
                                tunnel: w1025 -> [w1041]
                                i -> [w1044]
                                stop <- w1084 stop-if-true
                                w1049 = 3 ("index")
                                w1051 = 2 ("index")
                                w1053 = 1 ("index")
                                w1055 = 0 ("index")
                                w1082 = 2048 ("dimension size")
                                w1092 = 2048.0 ("element")
                                w1094 = T18 16 items=["<invalid type>"=0, "BYTE_IMG  (U8)"=8, "SHORT_IMG  (I16)"=16, "USHORT_IMG  (U16)"=20, "LONG_IMG  (I32)"=32, "ULONG_IMG  (U32)"=40, "FLOAT_IMG  (SGL)"=-32, "DOUBLE_IMG  (DBL)"=-64] ("image data type")
                                # "only the 1st fits file will have teliscope parameters"
                                n600 = Initialize Array(0.0 ("element"), w1082, w1082) -> (w1081:dbl[][])
                                n601 = for {
                                N: w1060 -> [_]
                                tunnel: w1111 -> [w1148]
                                shift-right: [w1143] -> w1109
                                shift-left: w1112 -> [w1149]
                                shift-right: [w1139] -> w1087
                                shift-left: w1110 -> [w1147]
                                shift-right: [w1134] -> w1108
                                shift-left: w1081 -> [w1130]
                                shift-right: [w1133] -> w1107
                                shift-left: w1081 -> [w1129]
                                shift-right: [w1132] -> w1106
                                shift-left: w1081 -> [w1128]
                                shift-right: [w1131] -> w1105
                                shift-left: w1081 -> [w1127]
                                tunnel: [w1126] -> w1042
                                n602 = flat-sequence {
                                tunnel: w1149 -> [w1159]
                                tunnel: w1148 -> [w1154]
                                tunnel: w1147 -> [w1158]
                                tunnel: [w1156] -> w1146
                                tunnel: [w1155] -> w1142
                                tunnel: [w1154] -> w1138
                                tunnel: [w1154] -> w1136
                                tunnel: [w1152] -> w1134
                                tunnel: w1130 -> [w1153]
                                tunnel: w1146 -> [w1170]
                                tunnel: [w1169] -> w1145
                                tunnel: w1142 -> [w1168]
                                tunnel: [w1167] -> w1141
                                tunnel: w1138 -> [w1166]
                                tunnel: [w1165] -> w1137
                                tunnel: w1136 -> [w1165]
                                tunnel: [w1162] -> w1133
                                tunnel: w1129 -> [w1163]
                                tunnel: w1145 -> [w1180]
                                tunnel: [w1179] -> w1144
                                tunnel: w1141 -> [w1178]
                                tunnel: [w1177] -> w1140
                                tunnel: w1137 -> [w1176]
                                tunnel: [w1176] -> w1135
                                tunnel: [w1173] -> w1132
                                tunnel: w1128 -> [w1174]
                                tunnel: w1144 -> [w1190]
                                tunnel: [w1189] -> w1143
                                tunnel: w1140 -> [w1188]
                                tunnel: [w1187] -> w1139
                                tunnel: w1135 -> [w1181]
                                tunnel: [w1184] -> w1131
                                tunnel: w1127 -> [w1185]
                                tunnel: [w1181] -> w1126
                                frame #0 {
                                n603 = call "grab image_2.vi"("ErrorIn"=w1158, "Image number"=u32 0, "BuffNr"=w1154, "ph"=w1159) -> ("output image"=w1151:dbl[][], "error out"=w1155:errorcluster, "hout"=w1156:u64)  [unwired: 4 in, 1 out]
                                n604 = To Extended Precision Float(1:w1151) -> (0:w1150:ext[][])
                                n605 = Add(x=w1150, y=w1153) -> (x+y=w1152:ext[][])
                                }
                                frame #1 {
                                n606 = call "grab image_2.vi"("ErrorIn"=w1168, "Image number"=u32 0, "BuffNr"=w1166, "ph"=w1170) -> ("output image"=w1161:dbl[][], "error out"=w1167:errorcluster, "hout"=w1169:u64)  [unwired: 4 in, 1 out]
                                n607 = To Extended Precision Float(1:w1161) -> (0:w1160:ext[][])
                                n608 = Add(x=w1160, y=w1163) -> (x+y=w1162:ext[][])
                                }
                                frame #2 {
                                n609 = call "grab image_2.vi"("ErrorIn"=w1178, "Image number"=u32 0, "BuffNr"=w1176, "ph"=w1180) -> ("output image"=w1172:dbl[][], "error out"=w1177:errorcluster, "hout"=w1179:u64)  [unwired: 4 in, 1 out]
                                n610 = To Extended Precision Float(1:w1172) -> (0:w1171:ext[][])
                                n611 = Add(x=w1171, y=w1174) -> (x+y=w1173:ext[][])
                                }
                                frame #3 {
                                n612 = call "grab image_2.vi"("ErrorIn"=w1188, "Image number"=u32 0, "BuffNr"=w1181, "ph"=w1190) -> ("output image"=w1183:dbl[][], "error out"=w1187:errorcluster, "hout"=w1189:u64)  [unwired: 4 in, 1 out]
                                n613 = To Extended Precision Float(1:w1183) -> (0:w1182:ext[][])
                                n614 = Add(x=w1182, y=w1185) -> (x+y=w1184:ext[][])
                                }
                                }
                                }
                                n615 = Format Into String(format string="%04d", w1044) -> (resulting string=w1039:string)  [unwired: 2 in, 1 out]
                                n616 = case shown="0, Default" w1041 {
                                tunnel: ["data_" "flat_"] -> w1038
                                frame 0, Default {
                                }
                                frame 1 {
                                }
                                }
                                n617 = Concatenate Strings(w1102, "\\" ("string"), w1038, w1039, ".fits" ("string")) -> (w1100:string)
                                n618 = String To Path(string=w1100) -> (path=w1099:path)
                                n619 = Divide(x=w1107, y=w1104) -> (x/y=w1078:ext[][])
                                n620 = Divide(x=w1106, y=w1104) -> (x/y=w1076:ext[][])
                                n621 = Divide(x=w1105, y=w1104) -> (x/y=w1074:ext[][])
                                n622 = Divide(x=w1108, y=w1104) -> (x/y=w1080:ext[][])
                                n623 = To Word Integer(number=w1078) -> (16bit integer=w1077:i16[][])
                                n624 = To Word Integer(number=w1076) -> (16bit integer=w1075:i16[][])
                                n625 = To Word Integer(number=w1074) -> (16bit integer=w1073:i16[][])
                                n626 = To Word Integer(number=w1080) -> (16bit integer=w1079:i16[][])
                                n627 = local write "CCD Display sp"(w1080) -> ()
                                n628 = local read "Exposure in msec"() -> (w1067:u32)
                                n629 = local read "End time Array"() -> (w1064:timestamp[])
                                n630 = Build Array(4.0 ("element"), w1092, w1092) -> (w1091:dbl[])
                                n631 = call "gfitsio-open-create-replace-file.vi"("advisory dialog? (display:T)"=FALSE, "function (open)"=T13."open or create", "file path (dialog if empty)"=w1099) -> ("error out"=w1096:errorcluster, "gfits refnum"=w1095:T19)  [unwired: 6 in, 1 out]
                                n632 = local read "Start time Array"() -> (w1066:timestamp[])
                                n633 = Build Array(w1079, w1077, w1075, w1073) -> (w1072:i16[][][])
                                n634 = Increment(x=w1044) -> (x+1=w1061:i32)
                                n635 = call "gfitsio-resize-image.vi"("image data type"=w1094, "naxes"=w1091, "error in (no error)"=w1096, "gfits refnum"=w1095) -> ("error out"=w1069:errorcluster, "dup gfits refnum"=w1071:T19)  [unwired: 6 in]
                                n636 = Index Array(array=w1064, index=w1061) -> (element=w1063:timestamp)
                                n637 = Index Array(array=w1066, index=w1061) -> (element=w1065:timestamp)
                                n638 = case shown="1, Default" w1044 {
                                tunnel: [TRUE FALSE] -> w1047
                                frame 0 {
                                }
                                frame 1, Default {
                                }
                                }
                                n639 = Index Array(array=w1045, index=w1055) -> (element=w1054:dbl)
                                n640 = Index Array(array=w1045, index=w1049) -> (element=w1048:dbl)
                                n641 = Index Array(array=w1045, index=w1053) -> (element=w1052:dbl)
                                n642 = Index Array(array=w1045, index=w1051) -> (element=w1050:dbl)
                                n643 = Index Array(array=w1046, index=w1051) -> (element=w1057:dbl)
                                n644 = Index Array(array=w1046, index=w1053) -> (element=w1058:dbl)
                                n645 = Index Array(array=w1046, index=w1055) -> (element=w1059:dbl)
                                n646 = Index Array(array=w1046, index=w1049) -> (element=w1056:dbl)
                                n647 = call "fits_header.vi"("gfits refnum"=w1071, "error in (no error)"=w1069, "start time"=w1065, "total scans"=w1062, "end time"=w1063, "Exposure"=w1067, "num of img added"=w1060, "lcvr1_2"=w1058, "lcvr2_4"=w1048, "lcvr1_4"=w1056, "lcvr2_2"=w1052, "lcvr1_1"=w1059, "lcvr1_3"=w1057, "lcvr2_1"=w1054, "lcvr2_3"=w1050, "Curr Scan"=w1061, "Teliscope parameters"=w1047) -> ("dup gfits refnum"=w1070:T19, "error out"=w1068:errorcluster)  [unwired: 9 in]
                                n648 = for {
                                N: 4 -> [_]
                                tunnel: w1072 -> [w1123] mode=indexing
                                shift-right: [w1122] -> w1090
                                shift-left: w1070 -> [w1125]
                                shift-right: [w1121] -> w1089
                                shift-left: w1068 -> [w1124]
                                i -> [w1120]
                                w1117 = 1.0 ("element")
                                n649 = Increment(x=w1120) -> (x+1=w1118:i32)
                                n650 = Build Array(w1118, w1117, w1117) -> (w1119:dbl[])
                                n651 = call "gfitsio-write-image-subset-i16-2d.vi"("fpixel"=w1119, "error in (no error)"=w1124, "data"=w1123, "gfits refnum"=w1125) -> ("error out"=w1121:errorcluster, "dup gfits refnum"=w1122:T19)  [unwired: 6 in]
                                }
                                n652 = call "gfitsio-close-file.vi"("error in (no error)"=w1089, "gfits refnum"=w1090) -> ("error out"=w1088:errorcluster, "Path"=w1085:path)  [unwired: 8 in]
                                n653 = Merge Errors(w1088, w1087) -> (w1086:errorcluster)
                                n654 = local write "Data is stored in the folder sp........."(w1085) -> ()
                                n655 = local read "Stop Spectroscopy sp"() -> (w1084:bool)
                              }
                            }
                            frame "Per Polarisation" {
                              n656 = local read "LCVR variable"() -> (w1195:T2)
                              n657 = Unbundle By Name(w1195) -> ("volt set of lcvr 1"=w1194:dbl[], "volt set of lcvr 2"=w1193:dbl[])
                              n658 = for {
                                N: w1198 -> [w1233]
                                tunnel: w1202 -> [w1268]
                                tunnel: w1201 -> [w1267]
                                shift-right: [w1266] -> w1200
                                shift-left: w1203 -> [w1269]
                                tunnel: w1199 -> [w1232]
                                tunnel: w1197 -> [w1253]
                                tunnel: [w1245] -> w1196
                                tunnel: w1194 -> [w1212]
                                tunnel: w1193 -> [w1211]
                                tunnel: [w1208] -> w1192
                                tunnel: w1191 -> [w1207]
                                i -> [w1210]
                                stop <- w1244 stop-if-true
                                w1254 = 2048.0 ("element")
                                w1256 = T18 16 items=["<invalid type>"=0, "BYTE_IMG  (U8)"=8, "SHORT_IMG  (I16)"=16, "USHORT_IMG  (U16)"=20, "LONG_IMG  (I32)"=32, "ULONG_IMG  (U32)"=40, "FLOAT_IMG  (SGL)"=-32, "DOUBLE_IMG  (DBL)"=-64] ("image data type")
                                n659 = Format Into String(format string="%04d", w1210) -> (resulting string=w1205:string)  [unwired: 2 in, 1 out]
                                n660 = for {
                                N: 4 -> [_]
                                tunnel: w1269 -> [w1294]
                                tunnel: w1268 -> [w1293]
                                shift-right: [w1291] -> w1246
                                shift-left: w1267 -> [w1292]
                                tunnel: [w1290] -> w1266
                                tunnel: w1232 -> [w1285]
                                tunnel: [w1284] -> w1251 mode=indexing
                                tunnel: [w1284] -> w1242
                                tunnel: [w1283] -> w1208
                                w1288 = 2048 ("dimension size")
                                n661 = Initialize Array(0.0 ("element"), w1288, w1288) -> (w1287:dbl[][])
                                n662 = for {
                                N: w1285 -> [_]
                                tunnel: w1294 -> [w1304]
                                tunnel: w1293 -> [w1295]
                                shift-right: [w1301] -> w1291
                                shift-left: w1292 -> [w1302]
                                shift-right: [w1298] -> w1286
                                shift-left: w1287 -> [w1296]
                                tunnel: [w1297] -> w1290
                                tunnel: [w1295] -> w1283
                                n663 = call "grab image_2.vi"("ErrorIn"=w1302, "Image number"=u32 0, "BuffNr"=w1295, "ph"=w1304) -> ("output image"=w1299:dbl[][], "error out"=w1301:errorcluster, "hout"=w1297:u64)  [unwired: 4 in, 1 out]
                                n664 = To Extended Precision Float(1:w1299) -> (0:w1300:ext[][])
                                n665 = Add(x=w1296, y=w1300) -> (x+y=w1298:ext[][])
                                }
                                n666 = Divide(x=w1286, y=w1285) -> (x/y=w1284:ext[][])
                                }
                                n667 = case shown="0, Default" w1207 {
                                tunnel: ["data_" "flat_"] -> w1204
                                frame 0, Default {
                                }
                                frame 1 {
                                }
                                }
                                n668 = Concatenate Strings(w1253, "\\" ("string"), w1204, w1205, ".fits" ("string")) -> (w1262:string)
                                n669 = String To Path(string=w1262) -> (path=w1261:path)
                                n670 = Build Array(4.0 ("element"), w1254, w1254) -> (w1252:dbl[])
                                n671 = call "gfitsio-open-create-replace-file.vi"("advisory dialog? (display:T)"=FALSE, "function (open)"=T13."open or create", "file path (dialog if empty)"=w1261) -> ("error out"=w1258:errorcluster, "gfits refnum"=w1257:T19)  [unwired: 6 in, 1 out]
                                n672 = local read "End time Array"() -> (w1235:timestamp[])
                                n673 = local read "Start time Array"() -> (w1237:timestamp[])
                                n674 = Increment(x=w1210) -> (x+1=w1230:i32)
                                n675 = local read "Exposure in msec"() -> (w1231:u32)
                                n676 = local write "CCD Display sp"(w1242) -> ()
                                n677 = call "gfitsio-resize-image.vi"("image data type"=w1256, "naxes"=w1252, "error in (no error)"=w1258, "gfits refnum"=w1257) -> ("error out"=w1239:errorcluster, "dup gfits refnum"=w1241:T19)  [unwired: 6 in]
                                n678 = To Word Integer(number=w1251) -> (16bit integer=w1250:i16[][][])
                                n679 = Index Array(array=w1237, index=w1230) -> (element=w1236:timestamp)
                                n680 = Index Array(array=w1235, index=w1230) -> (element=w1234:timestamp)
                                n681 = case shown="0" w1210 {
                                tunnel: [TRUE FALSE] -> w1213
                                frame 0 {
                                }
                                frame 1, Default {
                                }
                                }
                                n682 = Index Array(array=w1211, index=0) -> (element=w1220:dbl)
                                n683 = Index Array(array=w1212, index=2) -> (element=w1224:dbl)
                                n684 = Index Array(array=w1211, index=1) -> (element=w1218:dbl)
                                n685 = Index Array(array=w1212, index=1) -> (element=w1226:dbl)
                                n686 = Index Array(array=w1212, index=0) -> (element=w1228:dbl)
                                n687 = Index Array(array=w1212, index=3) -> (element=w1222:dbl)
                                n688 = Index Array(array=w1211, index=2) -> (element=w1216:dbl)
                                n689 = Index Array(array=w1211, index=3) -> (element=w1214:dbl)
                                n690 = call "fits_header.vi"("gfits refnum"=w1241, "error in (no error)"=w1239, "start time"=w1236, "total scans"=w1233, "end time"=w1234, "Exposure"=w1231, "num of img added"=w1232, "lcvr1_2"=w1226, "lcvr2_4"=w1214, "lcvr1_4"=w1222, "lcvr2_2"=w1218, "lcvr1_1"=w1228, "lcvr1_3"=w1224, "lcvr2_1"=w1220, "lcvr2_3"=w1216, "Curr Scan"=w1230, "Teliscope parameters"=w1213) -> ("dup gfits refnum"=w1240:T19, "error out"=w1238:errorcluster)  [unwired: 9 in]
                                n691 = for {
                                N: 4 -> [_]
                                tunnel: w1250 -> [w1282] mode=indexing
                                shift-right: [w1280] -> w1249
                                shift-left: w1240 -> [w1281]
                                shift-right: [w1278] -> w1248
                                shift-left: w1238 -> [w1279]
                                i -> [w1277]
                                w1275 = 1 ("element")
                                n692 = Increment(x=w1277) -> (x+1=w1276:i32)
                                n693 = Build Array(w1276, w1275, w1275) -> (w1274:i32[])
                                n694 = call "gfitsio-write-image-subset-i16-2d.vi"("fpixel"=w1274, "error in (no error)"=w1279, "data"=w1282, "gfits refnum"=w1281) -> ("error out"=w1278:errorcluster, "dup gfits refnum"=w1280:T19)  [unwired: 6 in]
                                }
                                n695 = call "gfitsio-close-file.vi"("error in (no error)"=w1248, "gfits refnum"=w1249) -> ("error out"=w1247:errorcluster, "Path"=w1243:path)  [unwired: 8 in]
                                n696 = Merge Errors(w1247, w1246) -> (w1245:errorcluster)
                                n697 = local write "Data is stored in the folder sp........."(w1243) -> ()
                                n698 = local read "Stop Spectroscopy sp"() -> (w1244:bool)
                              }
                            }
                          }
                          n699 = for {
                            N: w998 -> [_]
                            tunnel: w1015 -> [w1331]
                            shift-right: [w1328] -> w1017
                            shift-left: w1013 -> [w1330]
                            shift-right: [w1321] -> w1007
                            shift-left: timestamp[] [] -> [w1320]
                            shift-right: [w1319] -> w1008
                            shift-left: timestamp[] [] -> [w1318]
                            tunnel: w1002 -> [w1309]
                            tunnel: [w1308] -> w1000
                            tunnel: [w1307] -> w999
                            i -> [w1310]
                            stop <- w1329 stop-if-true
                            n700 = Increment(x=w1310) -> (x+1=w1327:i32)
                            n701 = local write "Steps performed sp"(w1327) -> ()
                            n702 = flat-sequence {
                              tunnel: w1309 -> [w1335]
                              tunnel: w1331 -> [w1336]
                              tunnel: w1330 -> [w1337]
                              tunnel: [w1337] -> w1324
                              tunnel: [w1336] -> w1323
                              tunnel: [w1335] -> w1322
                              tunnel: [w1333] -> w1321
                              tunnel: w1320 -> [w1332]
                              tunnel: [w1347] -> w1328
                              tunnel: w1324 -> [w1345]
                              tunnel: w1323 -> [w1346]
                              tunnel: w1322 -> [w1344]
                              tunnel: [w1500] -> w1319
                              tunnel: w1318 -> [w1499]
                              tunnel: w1326 -> [w1503]
                              tunnel: w1325 -> [w1508]
                              tunnel: [w1505] -> w1317
                              tunnel: [w1504] -> w1316
                              tunnel: [w1503] -> w1315
                              tunnel: [w1502] -> w1311
                              tunnel: w1317 -> [w1510]
                              tunnel: w1316 -> [w1509]
                              tunnel: w1315 -> [_]
                              tunnel: [w1510] -> w1314
                              tunnel: [w1509] -> w1313
                              tunnel: [w1511] -> w1312
                              tunnel: w1311 -> [w1511]
                              tunnel: w1314 -> [w1516]
                              tunnel: w1313 -> [w1514]
                              tunnel: w1312 -> [_]
                              tunnel: w1310 -> [_]
                              tunnel: [w1513] -> w1306
                              tunnel: [w1512] -> w1305
                              tunnel: [w1532] -> w1307
                              tunnel: [w1533] -> w1308
                              tunnel: w1306 -> [w1533]
                              tunnel: w1305 -> [w1532]
                              frame #0 {
                                n703 = Get Date/Time In Seconds() -> (seconds since 1Jan1904=w1334:timestamp)
                                n704 = Build Array (concatenate)(w1332, w1334) -> (w1333:timestamp[])
                              }
                              frame #1 {
                                n705 = local read "LCVR variable"() -> (w1342:T2)
                                n706 = Unbundle By Name(w1342) -> ("Open USB I/O Stuff"=w1338:T14, "volt set of lcvr 1"=w1341:dbl[], "volt set of lcvr 2"=w1340:dbl[])
                                n707 = call "version.vi"("USB Open Device Cluster"=w1338) -> ("Version"=w1339:dbl)  [unwired: 10 in]
                                n708 = case shown="\"Per scan\", Default" "Image averaging" {
                                tunnel: [w1352 w1429] -> w1347
                                tunnel: w1346 -> [w1354 w1428]
                                tunnel: w1345 -> [w1353 w1427]
                                tunnel: w1344 -> [w1355 w1426]
                                tunnel: w1338 -> [w1351 w1424]
                                tunnel: w1341 -> [w1350 w1423]
                                tunnel: w1340 -> [w1349 w1422]
                                tunnel: w1339 -> [w1348 w1421]
                                frame "Per scan", Default {
                                n709 = for {
                                N: w1355 -> [_]
                                tunnel: w1354 -> [w1363]
                                tunnel: w1353 -> [w1362]
                                tunnel: [w1361] -> w1352
                                tunnel: w1351 -> [w1360]
                                tunnel: w1350 -> [w1359]
                                tunnel: w1349 -> [w1358]
                                tunnel: w1348 -> [w1356]
                                stop <- w1357 stop-if-true
                                n710 = for {
                                N: 4 -> [_]
                                tunnel: w1363 -> [w1372]
                                tunnel: w1362 -> [w1371]
                                tunnel: [w1370] -> w1361
                                tunnel: w1360 -> [w1369]
                                tunnel: w1359 -> [w1368]
                                tunnel: w1358 -> [w1367]
                                tunnel: w1356 -> [w1366]
                                i -> [w1373]
                                n711 = flat-sequence {
                                tunnel: w1366 -> [w1377]
                                tunnel: w1367 -> [w1381]
                                tunnel: w1368 -> [w1382]
                                tunnel: w1369 -> [w1380]
                                tunnel: w1373 -> [w1384]
                                tunnel: w1373 -> [w1383]
                                tunnel: w1372 -> [w1399]
                                tunnel: w1371 -> [w1398]
                                tunnel: [w1397] -> w1365
                                tunnel: [w1419] -> w1370
                                tunnel: w1365 -> [w1419]
                                frame #0 {
                                # "simultaneous change in volt in two channels is not possible thus a frame sequence is put"
                                # "I found that this setteling time is nessary for proper polarimetry"
                                n712 = Index Array(array=w1382, index=w1383) -> (element=w1374:dbl)
                                n713 = Index Array(array=w1381, index=w1384) -> (element=w1378:dbl)
                                n714 = flat-sequence {
                                tunnel: [w1391] -> w1375
                                tunnel: w1374 -> [w1388]
                                tunnel: w1377 -> [w1390]
                                tunnel: 1 ("LC Channel") -> [w1389]
                                tunnel: w1374 -> [_]
                                tunnel: w1380 -> [w1391]
                                tunnel: w1377 -> [w1387]
                                tunnel: 2 ("LC Channel") -> [w1386]
                                tunnel: w1378 -> [w1385]
                                tunnel: w1375 -> [_]
                                frame #0 {
                                n715 = call "Meadowlark USB Set Voltage.VI"("LC Voltage"=w1385, "LC Channel"=w1386, "FW Version"=w1387, "USB Open Device Cluster"=w1391) -> ()  [unwired: 1 out]
                                n716 = call "Meadowlark USB Set Voltage.VI"("LC Voltage"=w1388, "LC Channel"=w1389, "FW Version"=w1390, "USB Open Device Cluster"=w1391) -> ()  [unwired: 1 out]
                                }
                                frame #1 {
                                n717 = Wait (ms)(milliseconds to wait=u32 100) -> ()  [unwired: 1 out]
                                }
                                }
                                }
                                frame #1 {
                                n718 = node-c288() -> (w1396:T9)  [unwired: 1 in]
                                n719 = timed-loop {
                                shift-right: [w1411] -> w1401
                                shift-left: w1399 -> [w1414]
                                shift-right: [w1412] -> w1400
                                shift-left: w1398 -> [w1413]
                                timing: w1396 -> [_]
                                timing-out: [_] -> w1395
                                stop <- w1410 continue-if-true
                                n720 = node-c288() -> ()  [unwired: 1 in, 1 out]
                                n721 = call <userlib>:"GetBusyStatus.vi"("error in (no error)"=w1413, "ph"=w1414) -> ("error out"=w1412:errorcluster, "BusyState"=w1410:bool, "hout"=w1411:u64)  [unwired: 2 in, 1 out]
                                n722 = node-c288() -> ()  [unwired: 1 in, 1 out]
                                }
                                n723 = node-c288(w1395) -> ()  [unwired: 1 out]
                                n724 = node-c288() -> (w1394:T9)  [unwired: 1 in]
                                n725 = timed-loop {
                                tunnel: w1401 -> [w1405]
                                shift-right: [w1402] -> w1397
                                shift-left: w1400 -> [w1403]
                                timing: w1394 -> [_]
                                timing-out: [_] -> w1393
                                stop <- w1404 stop-if-true
                                n726 = node-c288() -> ()  [unwired: 1 in, 1 out]
                                n727 = call <userlib>:"ForceTrigger.vi"("ph"=w1405, "error in (no error)"=w1403) -> ("Triggered"=w1404:bool, "error out"=w1402:errorcluster)  [unwired: 1 in, 2 out]
                                n728 = node-c288() -> ()  [unwired: 1 in, 1 out]
                                }
                                n729 = node-c288(w1393) -> ()  [unwired: 1 out]
                                }
                                frame #2 {
                                n730 = local read "Exposure in msec"() -> (w1420:u32)
                                n731 = Wait (ms)(milliseconds to wait=w1420) -> ()  [unwired: 1 out]
                                }
                                }
                                }
                                n732 = local read "Stop Spectroscopy sp"() -> (w1357:bool)
                                }
                                }
                                frame "Per Polarisation" {
                                n733 = for {
                                N: 4 -> [_]
                                tunnel: w1428 -> [w1436]
                                tunnel: w1426 -> [w1437]
                                shift-right: [w1435] -> w1429
                                shift-left: w1427 -> [w1434]
                                tunnel: w1424 -> [w1433]
                                tunnel: w1423 -> [w1432]
                                tunnel: w1422 -> [w1431]
                                tunnel: w1421 -> [w1430]
                                i -> [w1438]
                                n734 = flat-sequence {
                                tunnel: w1430 -> [w1442]
                                tunnel: w1431 -> [w1446]
                                tunnel: w1432 -> [w1447]
                                tunnel: w1433 -> [w1445]
                                tunnel: w1438 -> [w1448]
                                tunnel: w1437 -> [w1461]
                                tunnel: w1436 -> [w1460]
                                tunnel: [w1459] -> w1435
                                tunnel: w1434 -> [w1458]
                                frame #0 {
                                n735 = Index Array(array=w1446, index=w1448) -> (element=w1443:dbl)
                                n736 = Index Array(array=w1447, index=w1448) -> (element=w1440:dbl)
                                n737 = flat-sequence {
                                tunnel: [w1452] -> w1439
                                tunnel: w1443 -> [w1449]
                                tunnel: 2 ("LC Channel") -> [w1450]
                                tunnel: w1442 -> [w1451]
                                tunnel: w1445 -> [w1452]
                                tunnel: w1439 -> [w1456]
                                tunnel: w1442 -> [w1455]
                                tunnel: 1 ("LC Channel") -> [w1454]
                                tunnel: w1440 -> [w1453]
                                frame #0 {
                                n738 = call "Meadowlark USB Set Voltage.VI"("LC Voltage"=w1449, "LC Channel"=w1450, "FW Version"=w1451, "USB Open Device Cluster"=w1452) -> ()  [unwired: 1 out]
                                }
                                frame #1 {
                                n739 = call "Meadowlark USB Set Voltage.VI"("LC Voltage"=w1453, "LC Channel"=w1454, "FW Version"=w1455, "USB Open Device Cluster"=w1456) -> ()  [unwired: 1 out]
                                }
                                frame #2 {
                                n740 = Wait (ms)(milliseconds to wait=u32 100) -> ()  [unwired: 1 out]
                                }
                                }
                                }
                                frame #1 {
                                n741 = for {
                                N: w1461 -> [_]
                                tunnel: w1460 -> [w1468]
                                shift-right: [w1464] -> w1459
                                shift-left: w1458 -> [w1467]
                                stop <- w1463 stop-if-true
                                n742 = flat-sequence {
                                tunnel: w1468 -> [w1472]
                                tunnel: w1467 -> [w1471]
                                tunnel: [w1474] -> w1466
                                tunnel: [w1473] -> w1465
                                tunnel: w1466 -> [w1487]
                                tunnel: w1465 -> [w1486]
                                tunnel: [w1488] -> w1462
                                tunnel: [w1498] -> w1464
                                tunnel: w1462 -> [w1498]
                                frame #0 {
                                n743 = node-c288() -> (w1470:T9)  [unwired: 1 in]
                                n744 = timed-loop {
                                shift-right: [w1477] -> w1473
                                shift-left: w1471 -> [w1478]
                                tunnel: w1472 -> [w1479]
                                tunnel: [w1476] -> w1474
                                timing: w1470 -> [_]
                                timing-out: [_] -> w1469
                                stop <- w1475 continue-if-true
                                n745 = node-c288() -> ()  [unwired: 1 in, 1 out]
                                n746 = call <userlib>:"GetBusyStatus.vi"("error in (no error)"=w1478, "ph"=w1479) -> ("error out"=w1477:errorcluster, "BusyState"=w1475:bool, "hout"=w1476:u64)  [unwired: 2 in, 1 out]
                                n747 = node-c288() -> ()  [unwired: 1 in, 1 out]
                                }
                                n748 = node-c288(w1469) -> ()  [unwired: 1 out]
                                }
                                frame #1 {
                                n749 = node-c288() -> (w1485:T9)  [unwired: 1 in]
                                n750 = timed-loop {
                                tunnel: w1487 -> [w1492]
                                shift-right: [w1489] -> w1488
                                shift-left: w1486 -> [w1490]
                                timing: w1485 -> [_]
                                timing-out: [_] -> w1484
                                stop <- w1491 stop-if-true
                                n751 = node-c288() -> ()  [unwired: 1 in, 1 out]
                                n752 = call <userlib>:"ForceTrigger.vi"("ph"=w1492, "error in (no error)"=w1490) -> ("Triggered"=w1491:bool, "error out"=w1489:errorcluster)  [unwired: 1 in, 2 out]
                                n753 = node-c288() -> ()  [unwired: 1 in, 1 out]
                                }
                                n754 = node-c288(w1484) -> ()  [unwired: 1 out]
                                }
                                frame #2 {
                                n755 = local read "Exposure in msec"() -> (w1497:u32)
                                n756 = Wait (ms)(milliseconds to wait=w1497) -> ()  [unwired: 1 out]
                                }
                                }
                                n757 = local read "Stop Spectroscopy sp"() -> (w1463:bool)
                                }
                                }
                                }
                                }
                                }
                                }
                              }
                              frame #2 {
                                n758 = Get Date/Time In Seconds() -> (seconds since 1Jan1904=w1501:timestamp)
                                n759 = Build Array (concatenate)(w1499, w1501) -> (w1500:timestamp[])
                              }
                              frame #3 {
                                n760 = Unbundle By Name(w1508) -> ("VISA resource name"=w1507:refnum<visa-resource-name>, "Axis 2"=w1504:u32, "Rotate in deg 2"=w1502:dbl, "Error In"=w1506:errorcluster)
                                n761 = call <userlib>:"Move Relative.vi"("error in (no error)"=w1506, "Position (0 units)"=w1502, "Axis (1)"=w1504, "VISA resource name"=w1507) -> ("VISA resource name out"=w1505:refnum<visa-resource-name>)  [unwired: 2 in, 1 out]
                              }
                              frame #4 {
                              }
                              frame #5 {
                                n762 = node-c288() -> (w1518:T9)  [unwired: 1 in]
                                n763 = timed-loop {
                                tunnel: w1516 -> [w1526]
                                tunnel: w1514 -> [w1519]
                                shift-right: [w1524] -> _
                                shift-left: 1000.0 ("Position (units)") -> [w1525]
                                timing: w1518 -> [_]
                                timing-out: [_] -> w1517
                                tunnel: [w1520] -> w1513
                                tunnel: [w1519] -> w1512
                                stop <- w1521 stop-if-true
                                n764 = node-c288() -> ()  [unwired: 1 in, 1 out]
                                n765 = call <userlib>:"Read Actual Position.vi"("Axis (1)"=w1519, "VISA resource name"=w1526) -> ("Position (units)"=w1524:dbl, "VISA resource name out"=w1520:refnum<visa-resource-name>)  [unwired: 3 in, 1 out]
                                n766 = Subtract(x=w1525, y=w1524) -> (x-y=w1523:dbl)
                                n767 = Equal?(x=w1523, y=0.0) -> (x = y?=w1521:bool)
                                n768 = node-c288() -> ()  [unwired: 1 in, 1 out]
                                }
                                n769 = node-c288(w1517) -> ()  [unwired: 1 out]
                              }
                              frame #6 {
                                # "I am forced to use this delay\nas my motor has very bad settling \ntime"
                                n770 = Wait (ms)(milliseconds to wait=u32 5000) -> ()  [unwired: 1 out]
                              }
                            }
                            n771 = local read "Exposure in msec"() -> (w1326:u32)
                            n772 = local read "Motor Variable"() -> (w1325:T5)
                            n773 = local read "Stop Spectroscopy sp"() -> (w1329:bool)
                          }
                          "End time Array" <- w1008
                          "Start time Array" <- w1007
                        }
                        frame #1 {
                          n774 = case shown="0, Default" w1534 {
                            tunnel: [w1543 FALSE ("T button?")] -> w1538
                            frame 0, Default {
                              n775 = Two Button Dialog(message="Going for flat field. If yes move\nteliscope to quiet sun and start \nmoving it before clicking on \"yes\"", 1:"No" ("F button name (\"Cancel\")"), 2:"Yes" ("T button name (\"OK\")")) -> (T button?=w1543:bool)
                            }
                            frame 1 {
                            }
                          }
                          n776 = local read "Stop Spectroscopy sp"() -> (w1540:bool)
                          n777 = Not(x=w1540) -> (.not. x?=w1539:bool)
                          n778 = And(x=w1539, y=w1538) -> (x .and. y?=w1537:bool)
                        }
                        frame #2 {
                          n779 = case shown="0, Default" w1548 {
                            tunnel: w1550 -> [w1568 w1578]
                            tunnel: w1549 -> [w1567 w1577]
                            frame 0, Default {
                              # "This gives mid point"
                              n780 = local read "initial absolute position"() -> (w1562:dbl)
                              n781 = local read "Motor Variable"() -> (w1566:T5)
                              n782 = Unbundle By Name(w1566) -> ("Rotate in deg 2"=w1558:dbl)
                              n783 = local read "Scan steps sp"() -> (w1561:dbl)
                              n784 = Divide(x=w1561, y=10.0) -> (x/y=w1559:dbl)
                              n785 = Multiply(x=w1559, y=w1558) -> (x*y=w1557:dbl)
                              n786 = Divide(x=w1557, y=2.0) -> (x/y=w1554:dbl)
                              n787 = Multiply(x=w1558, y=w1561) -> (x*y=w1565:dbl)
                              n788 = Divide(x=w1565, y=2.0) -> (x/y=w1563:dbl)
                              n789 = Add(x=w1563, y=w1562) -> (x+y=w1555:dbl)
                              n790 = Subtract(x=w1555, y=w1554) -> (x-y=w1553:dbl)
                              n791 = call <userlib>:"Move Absolute.vi"("Position (0 units)"=w1553, "Axis (1)"=w1567, "VISA resource name"=w1568) -> ()  [unwired: 3 in, 2 out]
                            }
                            frame 1 {
                              n792 = local read "initial absolute position"() -> (w1570:dbl)
                              n793 = local read "Motor Variable"() -> (w1576:T5)
                              n794 = Unbundle By Name(w1576) -> ("Rotate in deg 2"=w1575:dbl)
                              n795 = local read "Scan steps sp"() -> (w1574:dbl)
                              n796 = Multiply(x=w1575, y=w1574) -> (x*y=w1573:dbl)
                              n797 = Divide(x=w1573, y=2.0) -> (x/y=w1571:dbl)
                              n798 = Add(x=w1571, y=w1570) -> (x+y=w1569:dbl)
                              n799 = call <userlib>:"Move Absolute.vi"("Position (0 units)"=w1569, "Axis (1)"=w1577, "VISA resource name"=w1578) -> ()  [unwired: 3 in, 2 out]
                            }
                          }
                        }
                      }
                    }
                  }
                  frame #4 {
                    n800 = Merge Errors(w1585, w1582) -> (w1584:errorcluster)
                    n801 = local read "Stop Spectroscopy sp"() -> (w1583:bool)
                    n802 = call <vilib>:"Simple Error Handler.vi"("error in (no error)"=w1584) -> ()  [unwired: 4 in, 5 out]
                    n803 = case shown="False" w1583 {
                      tunnel: w1581 -> [w1588 _]
                      tunnel: w1580 -> [w1587 _]
                      tunnel: w1579 -> [w1586 _]
                      frame False {
                        n804 = flat-sequence {
                          tunnel: w1588 -> [w1595]
                          tunnel: w1587 -> [w1594]
                          tunnel: w1586 -> [w1593]
                          frame #0 {
                            n805 = Two Button Dialog(message="Perform polarisation calibration of beam\npath after teliscope ? ", 1:"NO" ("F button name (\"Cancel\")"), 2:"YES" ("T button name (\"OK\")")) -> (T button?=w1589:bool)
                            n806 = case shown="True" w1589 {
                              tunnel: w1595 -> [_ w1599]
                              tunnel: w1594 -> [_ w1598]
                              tunnel: w1593 -> [_ w1597]
                              frame False {
                              }
                              frame True {
                                n807 = local read "LCVR variable"() -> (w1596:T2)
                                n808 = call "polcal_new.vi"("LCVR variable"=w1596, "file path (dialog if empty)"=w1598, "BuffNr"=w1597, "ph"=w1599) -> ()  [unwired: 6 in, 2 out]
                              }
                            }
                          }
                          frame #1 {
                            n809 = Two Button Dialog(message="Spectropolarimetry completed successfully!!.    Reset Motor?", 1:"No" ("button name (\"OK\")"), 2:"Yes" ("T button name (\"OK\")")) -> (T button?=w1600:bool)
                            n810 = case shown="True" w1600 {
                              frame False {
                              }
                              frame True {
                                n811 = local read "Motor Variable"() -> (w1608:T5)
                                n812 = Unbundle By Name(w1608) -> ("VISA resource name"=w1607:refnum<visa-resource-name>, "Axis 2"=w1606:u32, "Error In"=w1605:errorcluster)
                                n813 = local read "initial absolute position"() -> (w1604:dbl)
                                n814 = call <userlib>:"Move Absolute.vi"("error in (no error)"=w1605, "Position (0 units)"=w1604, "Axis (1)"=w1606, "VISA resource name"=w1607) -> ()  [unwired: 2 in, 2 out]
                              }
                            }
                          }
                        }
                      }
                      frame True {
                        n815 = local write "Stop Spectroscopy sp"(FALSE ("Stop Spectroscopy sp")) -> ()
                        n816 = Two Button Dialog(message="Spectropolarimetry Stopped by user. Reset motor?", 1:"No" ("F button name (\"Cancel\")"), 2:"Yes" ("T button name (\"OK\")")) -> (T button?=w1610:bool)
                        n817 = case shown="True" w1610 {
                          frame False {
                          }
                          frame True {
                            n818 = local read "Motor Variable"() -> (w1618:T5)
                            n819 = Unbundle By Name(w1618) -> ("VISA resource name"=w1617:refnum<visa-resource-name>, "Axis 2"=w1616:u32, "Error In"=w1615:errorcluster)
                            n820 = local read "initial absolute position"() -> (w1614:dbl)
                            n821 = call <userlib>:"Move Absolute.vi"("error in (no error)"=w1615, "Position (0 units)"=w1614, "Axis (1)"=w1616, "VISA resource name"=w1617) -> ()  [unwired: 2 in, 2 out]
                          }
                        }
                      }
                    }
                  }
                }
                n822 = Bundle By Name(cluster=w796, "Open USB I/O Stuff"=w795, "Current Lcvr Temp"=w793) -> (w794:T2)
                n823 = local write "LCVR variable"(w794) -> ()
              }
            }
          }
          frame True {
          }
        }
      }
      n824 = property on="LCVR Temperature in deg C\n      Set         Current" class="Arr (strict)"("Value"=w344) -> ()  [unwired: 2 in, 2 out]
    }
    frame #3 {
      n825 = local read "Cam Variable"() -> (w1638:T6)
      n826 = local read "Motor Variable"() -> (w1634:T5)
      n827 = Unbundle By Name(w1638) -> ("hout"=w1637:u64)
      n828 = Unbundle By Name(w1634) -> ("VISA resource name"=w1633:refnum<visa-resource-name>, "Axis 2"=w1628:u32)
      n829 = call <userlib>:"CancelImages.vi"("ph"=w1637) -> ("error out"=w1636:errorcluster, "ErrorCode"=w1635:i32)  [unwired: 2 in, 1 out]
      n830 = call <vilib>:"Simple Error Handler.vi"("error code (no error:0)"=w1635, "error in (no error)"=w1636) -> ()  [unwired: 3 in, 5 out]
      n831 = call <userlib>:"Search For Home.vi"("Home mode"=T8."Find Home Signal", "Axis (1)"=w1628, "VISA resource name"=w1633) -> ("VISA resource name out"=w1631:refnum<visa-resource-name>)  [unwired: 4 in, 1 out]
      n832 = local read "LCVR closing\nvariable"() -> (w1639:T1)
      n833 = node-c288() -> (w1630:T9)  [unwired: 1 in]
      n834 = timed-loop {
        timing: w1630 -> [_]
        timing-out: [_] -> w1629
        tunnel: w1631 -> [w1645]
        tunnel: w1628 -> [w1644]
        tunnel: [w1642] -> w1626
        stop <- w1643 stop-if-true
        n835 = node-c288() -> ()  [unwired: 1 in, 1 out]
        n836 = call <userlib>:"Get Axis Motion Status.vi"("Axis (1)"=w1644, "VISA resource name"=w1645) -> ("Motion Done"=w1643:bool, "VISA resource name out"=w1642:refnum<visa-resource-name>)  [unwired: 3 in, 1 out]
        n837 = node-c288() -> ()  [unwired: 1 in, 1 out]
      }
      n838 = call "Meadowlark USB Easy Close.vi"("USB Device and Pipes Array"=w1639) -> ()
      n839 = flat-sequence {
        tunnel: w1626 -> [w1641]
        tunnel: [w1641] -> w1625
        frame #0 {
          n840 = Wait (ms)(milliseconds to wait=u32 3000) -> ()  [unwired: 1 out]
        }
        frame #1 {
        }
      }
      n841 = call <userlib>:"Enable Disable Motor.vi"("Action (F - OFF)"=FALSE, "Axis (1)"=w1628, "VISA resource name"=w1625) -> ()  [unwired: 3 in, 2 out]
      n842 = node-c288(w1629) -> ()  [unwired: 1 out]
    }
  }
  n843 = property on="CCD Display" class="IntGraph (strict)"("XScale.Minimum"=w4) -> ()  [unwired: 2 in, 2 out]
  n844 = property on="CCD Display" class="IntGraph (strict)"("YScale.Minimum"=w4) -> ()  [unwired: 2 in, 2 out]
  n845 = property on="Finish" class="Bool"("Visible"=w1) -> ()  [unwired: 2 in, 2 out]
  n846 = property on="Slide" class="Slide (strict)"("Visible"=w1) -> ()  [unwired: 2 in, 2 out]
  n847 = property on="Slide sp" class="Slide (strict)"("Visible"=w1) -> ()  [unwired: 2 in, 2 out]
  n848 = property on="Status" class="Str"("Visible"=w1) -> ()  [unwired: 2 in, 2 out]
  n849 = property on="Apply" class="Bool (strict)"("Visible"=w1) -> ()  [unwired: 2 in, 2 out]
  n850 = property on="initial absolute position" class="DigNum (strict)"("Visible"=w1) -> ()  [unwired: 2 in, 2 out]
  n851 = property on="CCD Display" class="IntGraph (strict)"("YScale.Maximum"=w3) -> ()  [unwired: 2 in, 2 out]
  n852 = property on="CCD Display" class="IntGraph (strict)"("XScale.Maximum"=w3) -> ()  [unwired: 2 in, 2 out]
  n853 = property on="Voltage-Retardance file path for lcvr2" class="Path"("Visible"=w1) -> ()  [unwired: 2 in, 2 out]
  n854 = property on="Rotate in deg" class="DigNum (strict)"("Visible"=w1) -> ()  [unwired: 2 in, 2 out]
  n855 = property on="VISA Refnum in" class="VISAName"("Visible"=w1) -> ()  [unwired: 2 in, 2 out]
  n856 = property on="CONTROLLER Number" class="Str"("Visible"=w1) -> ()  [unwired: 2 in, 2 out]
  n857 = property on="Axis" class="DigNum (strict)"("Visible"=w1) -> ()  [unwired: 2 in, 2 out]
  n858 = property on="Initialise Device" class="Ring (strict)"("Visible"=w1) -> ()  [unwired: 2 in, 2 out]
  n859 = property on="Close USO software" class="Bool (strict)"("Visible"=w1) -> ()  [unwired: 2 in, 2 out]
  n860 = property on="accept intensity" class="Bool (strict)"("Visible"=w1) -> ()  [unwired: 2 in, 2 out]
  n861 = property on="LCVR Set Temperature" class="DigNum (strict)"("Visible"=w1) -> ()  [unwired: 2 in, 2 out]
  n862 = property on="Voltage-Retardance file path for lcvr1" class="Path"("Visible"=w1) -> ()  [unwired: 2 in, 2 out]
  n863 = property on="accept intensity sp" class="Bool (strict)"("Visible"=w1) -> ()  [unwired: 2 in, 2 out]
  n864 = property on="Start observation session" class="Bool (strict)"("Visible"=w1) -> ()  [unwired: 2 in, 2 out]
  n865 = property on="Delay in msec" class="DigNum (strict)"("Visible"=w1) -> ()  [unwired: 2 in, 2 out]
  n866 = property on="Exposure in msec" class="DigNum (strict)"("Visible"=w1) -> ()  [unwired: 2 in, 2 out]
  n867 = property on="InterfaceType" class="Ring (strict)"("Visible"=w1) -> ()  [unwired: 2 in, 2 out]
  n868 = property on="spectroscopy/spectropolarimetry tab" class="TabCtl (strict)"("Visible"=w1) -> ()  [unwired: 2 in, 2 out]
  "Buf no 2" <- w2
  "Buf no 1" <- w2
